vi "RotinaEnsaio.vi"() -> ()   [LabVIEW 2019]
uses:
  <vilib>/Platform/TimedLoop/XDataNode/timing_clust.ctl
  <vilib>/Platform/TimedLoop/XDataNode/nitl_modes.ctl
  <vilib>/Platform/TimedLoop/XDataNode/wakeup.ctl
  <vilib>/DAQmx/write.llb/DAQmx Write (Digital Bool 1Line 1Point).vi
  <vilib>/DAQmx/write.llb/DAQmx Write (Analog DBL 1Chan 1Samp).vi
  <vilib>/Analysis/5stat.llb/RMS (DBL).vi
  <vilib>/DAQmx/write.llb/DAQmx Write (Counter Frequency 1Chan 1Samp).vi
  <vilib>/DAQmx/create/channels.llb/DAQmx Create Channel (DO-Digital Output).vi
  <vilib>/DAQmx/miscellaneous.llb/DAQmx Fill In Error Info.vi
  FPGA_RW_Vars.vi
  <vilib>/DAQmx/create/channels.llb/DAQmx Create Channel (AO-Voltage-Basic).vi
  <vilib>/DAQmx/create/channels.llb/DAQmx Create Channel (CO-Pulse Generation-Frequency).vi
  <vilib>/DAQmx/configure/timing.llb/DAQmx Timing (Implicit).vi
  <vilib>/addons/control/pid/pid.llb/PID Advanced (DBL).vi
  <vilib>/Waveform/WDTFileIO.llb/ Write Waveform to File.vi
  <vilib>/Waveform/WDTFileIO.llb/ Write Waveforms to File (1D).vi
  <vilib>/Platform/TimedLoop/XDataNode/XDataNode.xnode
  <vilib>/addons/control/pid/NI_PID_pid.lvlib
  <vilib>/Analysis/NI_AALPro.lvlib
  <resource>/objmgr/daqmx.rc
  <vilib>/Platform/TimedLoop/XDataNode/XDNodeRunTimeDep.lvlib
  <vilib>/Analysis/NI_AALBase.lvlib
  <instrlib>/Yokogawa WT100 Series/Yokogawa WT100 Series.lvlib
panel:
  in  "error in 2":errorcluster caption="error in"
  in  "error in":errorcluster
  out "Tempo de Ensaio":string
  out "Erro Valv. Sucção":errorcluster
  out "Erro Pressão":errorcluster
  out "Erro Fluximetro":errorcluster
  in  "Ativar Compressor?":bool
  in  "Tab Control":T1(tab)
  in  "Temp. Suc. Auto?":bool
  in  "Setpoint T. Suc. [ºC]":dbl=60.0
  out "Duty Cycle da Resistência [%] 2":dbl min=0.0 max=100.0
  in  "DC da Resistência (Suc) [%]":dbl min=0.0 max=100.0
  out "GE Comp S [bar]":dbl
  out "GE Valv S [bar]":dbl
  out "RMS Inferior [g]":dbl
  out "RMS Bancada [g]":dbl
  out "RMS Superior [g]":dbl
  out "Grafico Vibração":T2(graph)
  out "Grafico Pressão":T3(graph)
  out "Tensão da válvula de sucção [V]":dbl min=0.0 max=100.0
  out "Duty Cycle da Resistência [%]":dbl min=0.0 max=100.0
  out "Setpoint da abertura da valvula":dbl=3720000.0
  out "Velocidade do motor de descarga":dbl
  in  "Tensão da válvula de sucção [V]":dbl=0.2 min=0.0 max=100.0
  out "Vazão Mássica [kg/h]":dbl
  in  "Ativar Ventilador?":bool=TRUE
  in  "P. Sucção Auto?":bool
  in  "Setpoint Sucção [bar]":dbl=0.626
  out "Descarga [bar]":dbl
  out "Sucção [bar]":dbl
  in  "Setpoint T. Desc. [ºC]":dbl=60.0
  in  "Temp. Desc. Auto?":bool
  out "Corrente RMS [A] (LEM)":dbl
  out "Descarga [ºC]":dbl
  out "Sucção [ºC]":dbl
  out "Grafico Temperatura":T4(graph)
  out "Bobina 2 [ºC]":dbl
  in  "DC da Resistência (Des) [%]":dbl min=0.0 max=100.0
  in  "Abertura da válvula de descarga":dbl=16000.0 format="%#_10f"
  in  "Velocidade do motor de descarga":dbl
  out "Grafico Corrente":T5(graph)
  out "Grafico Vazão":dbl(graph)
  out "Posição Atual da Válvula de Descarga":dbl format="%#_9f"
  out "Intermed [bar]":dbl
  in  "Vel. Valv. Desc. Auto?":bool=TRUE
  in  "P. Descarga Auto?":bool
  in  "Setpoint Descarga [bar]":dbl=7.616
  out "Abertura Atual da Válvula de Descarga":dbl format="%#_9f"
  out "Corrente RMS [A] (WT130)":dbl
  out "Tensão RMS [V] (WT130)":dbl
  out "Potência [W] (WT130)":dbl
  out "Corrente RMS [A] (TMCS)":dbl
  out "Bobina 1 [ºC]":dbl
  out "Tensão RMS [V] (DAQ)":dbl
  out "Corpo [ºC]":dbl
  out "Ambiente [ºC]":dbl
  out "Reservatório [ºC]":dbl
  in  "Unidade Pressão":T6(ring)
  in  "Eixo X":u16(ring) items=["Amostras", "Tempo [s]", "Tempo [min]", "Tempo [h]"]
  out "T.S. Auto?":bool
  in  "Ganhos - Temperatura Sucção":T7={"proportional gain (Kc)"=0.1, "integral time (Ti, min)"=30.0, "derivative time (Td, min)"=0.5} {"derivative time (Td, min)" format="%#_10g"; "integral time (Ti, min)" format="%#_10g"; "proportional gain (Kc)" format="%#_10g"}
  in  "Frequência PWM [Hz]":dbl=2.0 min=1e-12
  in  "Pasta do projeto":path=path "D:/Documentos/Amaciamento/Resultados/TESTE"
  out "dt - Leitura Temperatura [s]":dbl
  out "dt - At PressãoTemp/Le Pos":dbl
  out "dt - Leitura Fluxímetro [s]":dbl
  out "dt - Salvar dados [s]":dbl
  out "dt - Atualiza Gráficos [s]":dbl
  in  "Nome de Base do Arquivo - Geral":string="medicoesGerais"
  in  "Limite inferior da posição da válvula":dbl=3698950.0 format="%#_10f"
  out "T.D. Auto?":bool
  out "P. S. Auto?":bool
  out "P. D. Auto?":bool
  in  "Ganhos - Pressão de Descarga":T7={"proportional gain (Kc)"=-6000.0, "integral time (Ti, min)"=0.5, "derivative time (Td, min)"=0.0} {"derivative time (Td, min)" format="%#_10g"; "integral time (Ti, min)" format="%#_10g"; "proportional gain (Kc)" format="%#_10g"}
  out "Vel. M. Auto?":bool
  in  "Ganhos - Posição do motor":T7={"proportional gain (Kc)"=-0.27, "integral time (Ti, min)"=0.0, "derivative time (Td, min)"=0.0} {"derivative time (Td, min)" format="%#_10g"; "integral time (Ti, min)" format="%#_10g"; "proportional gain (Kc)" format="%#_10g"}
  in  "Ganhos - Pressão de Sucção":T7={"proportional gain (Kc)"=2.0, "integral time (Ti, min)"=0.2, "derivative time (Td, min)"=0.0} {"derivative time (Td, min)" format="%#_10g"; "integral time (Ti, min)" format="%#_10g"; "proportional gain (Kc)" format="%#_10g"}
  in  "Ganhos - Temperatura Descarga":T7={"proportional gain (Kc)"=0.1, "integral time (Ti, min)"=30.0, "derivative time (Td, min)"=0.5} {"derivative time (Td, min)" format="%#_10g"; "integral time (Ti, min)" format="%#_10g"; "proportional gain (Kc)" format="%#_10g"}
  in  "Limites de velocidade":T8={"Velocidade Máxima"=10000.0, "Velocidade Mínima"=-10000.0}
  in  "Nome de Base do Arquivo - Vibração":string="vib"
  in  "Nome de Base do Arquivo - Corrente":string="corr"
  out "dt - Controle Pressão [s]":dbl
  in  "Limite Superior DC Auto [%]":dbl=60.0 format="%#_13g"
  in  "Limite inferior - Válvula de sucção":dbl=0.18 format="%#_13g"
  in  "Nome de Base do Arquivo - Tensão":string="ten"
  out "G Temperaturas":T4(graph)
  out "G Pressão de Descarga":T9(graph)
  out "G Pressão de Sucção":T10(graph)
  out "G Corrente RMS":T5(graph)
  out "G Pressão Intermed":dbl(graph)
  out "G Vazão":dbl(graph)
  out "G Vel. do Motor da Válvula de Descarga":dbl(graph)
  out "G Posição do Encoder":T11(graph)
  out "G Tensão na válvula de Sucção":dbl(graph)
  out "Erro FPGA":errorcluster
  out "G Potência Yokogawa":dbl(graph)
  out "DC":dbl(graph)
  out "Error Out":errorcluster
  out "G Tensão Yokogawa":dbl(graph)
  out "Erro Motor":errorcluster
  out "error out":errorcluster
  out "Acc":dbl[](array[numeric])
  in  "STOP":bool
  in  "Limpar Gráficos":bool
  # "Isobutano (R600a):\n\n-23,3/54,4 -> 0,626/7,616\n-17,5/90    -> 0,8012/16,4073\n-10/100     -> 1,08127/19,8569\n\nR134a\n\n -23,3/54,4 -> 1,148/14,698"
  # "Pressão"
  # "Temperatura"
  # "Corrente"
  # "Vazão"
  # "Vibração"
  # "Controle Manual"
  # "Controle Aplicado"
  # "PID"
  # "Ranges"
  # "Arquivos"
  # "Resistência"
  # "Loops"
  # "Gráficos"
  # "Identificação de sistemas"
  # "Erros"
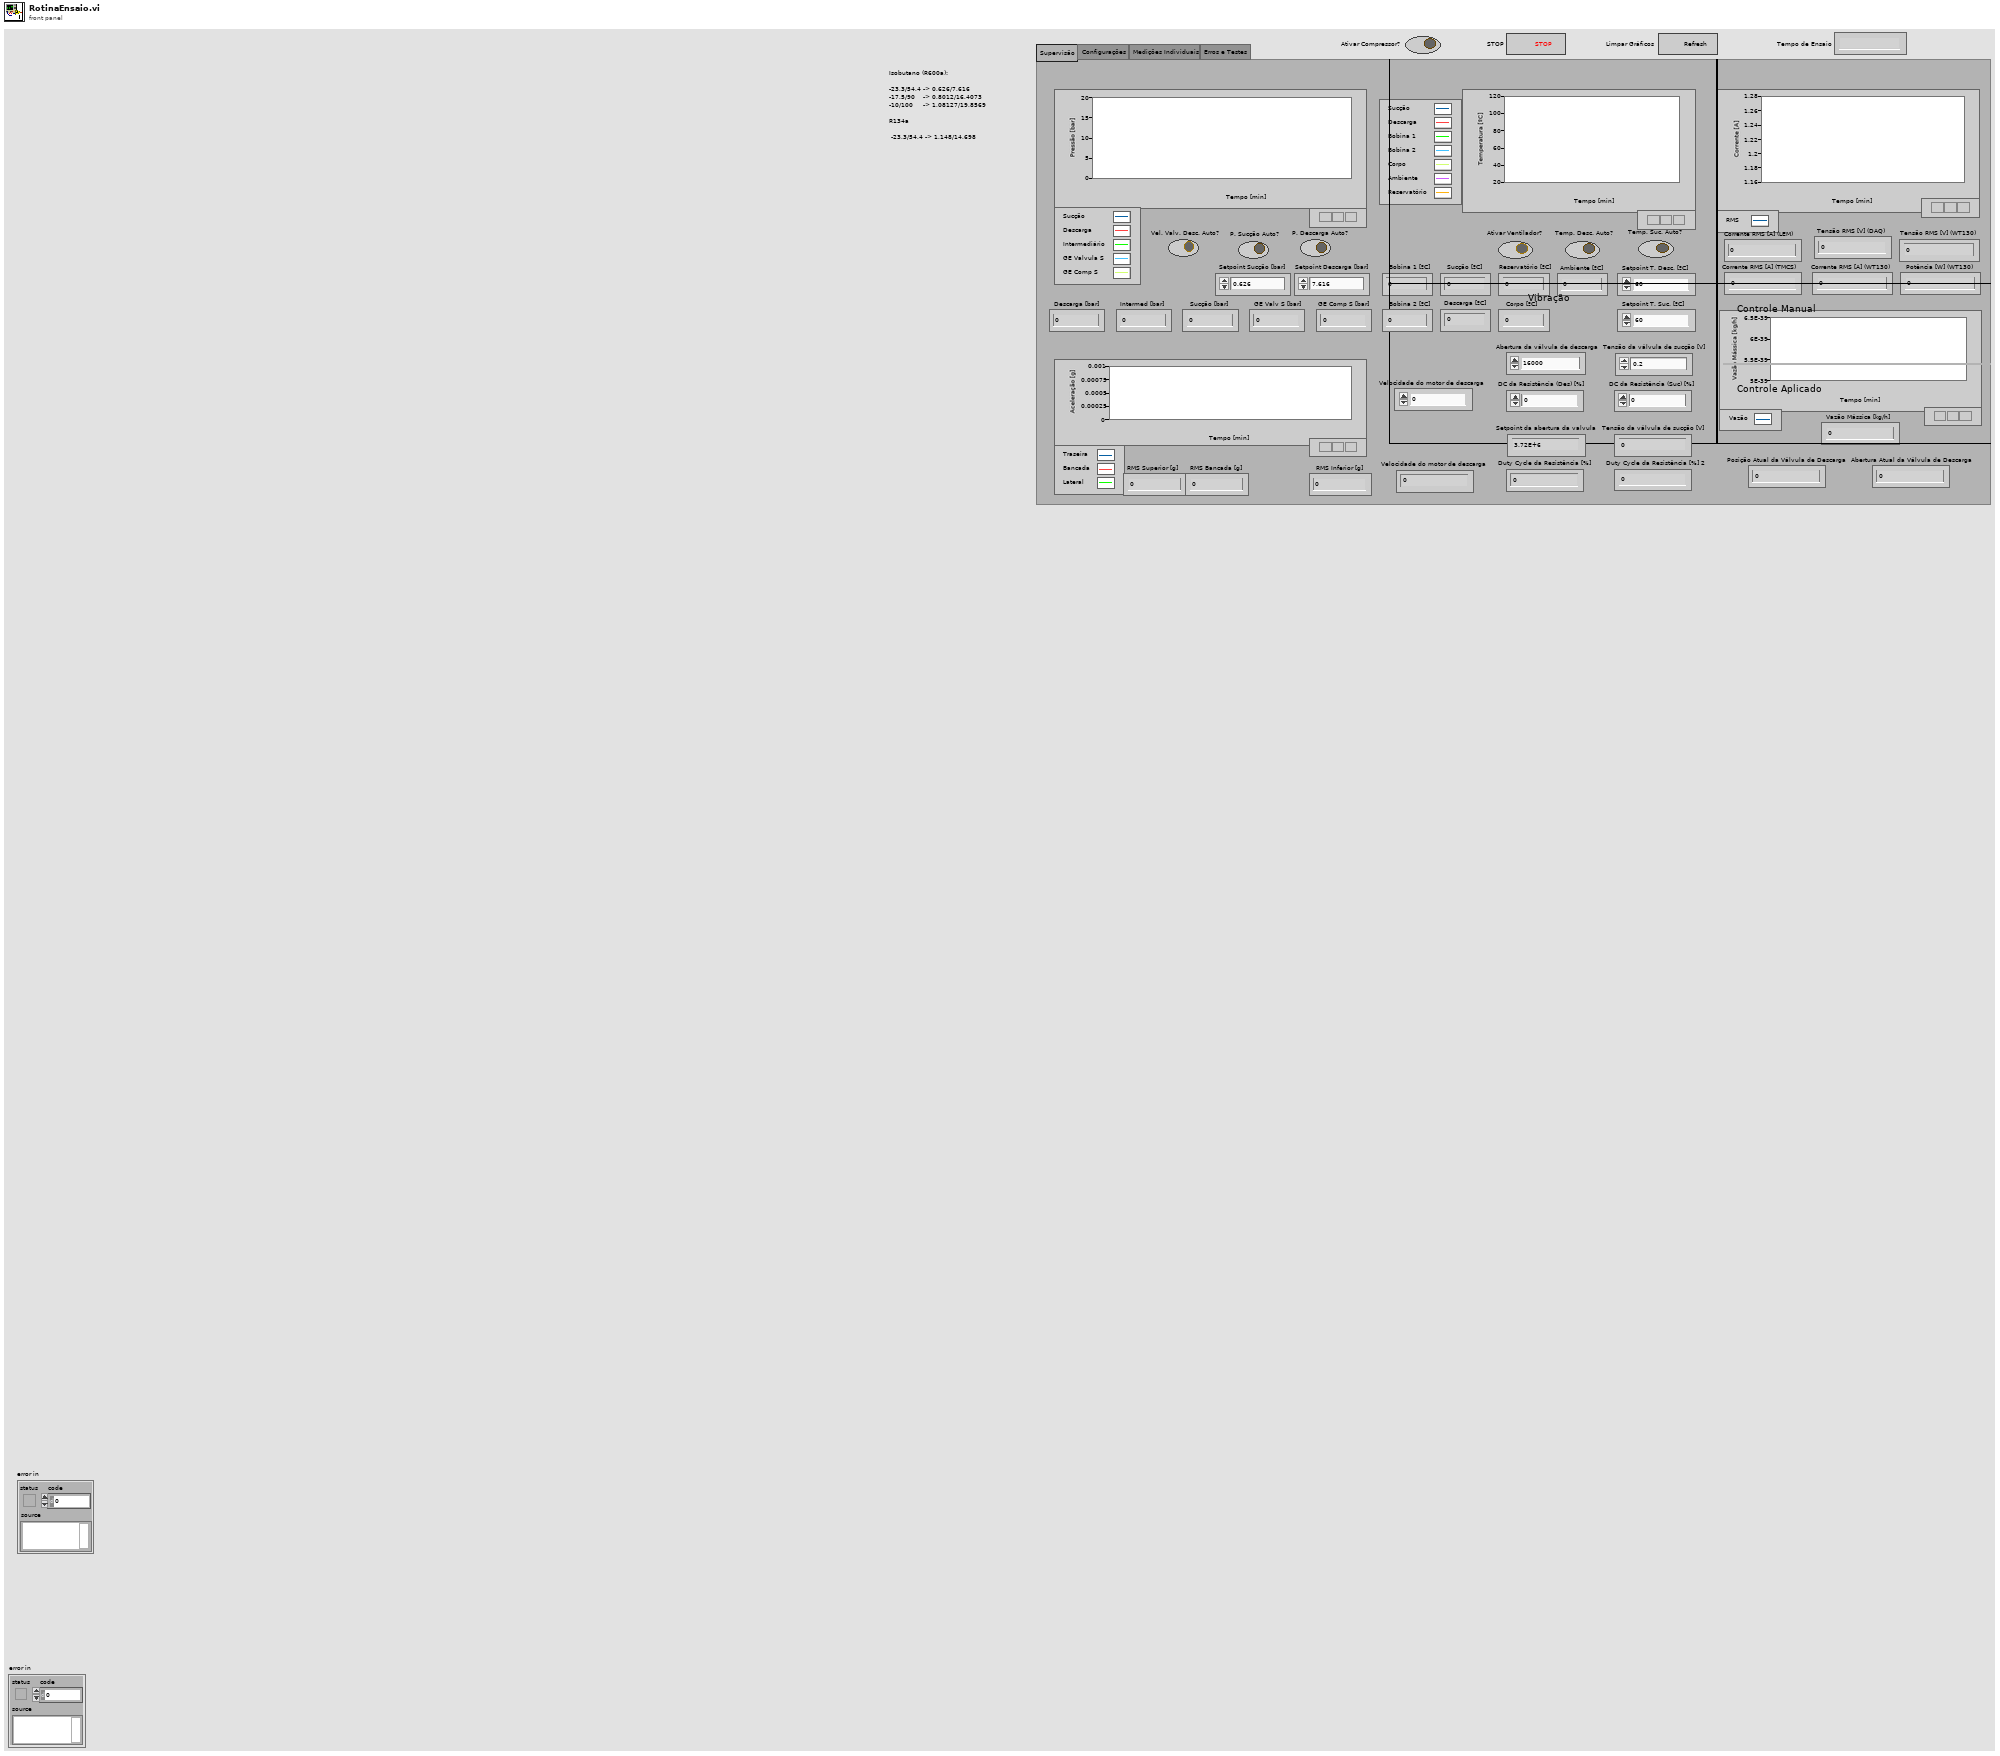
[diagram p1: front panel]
types:
  T1 = enum32{"Supervisão", "Configurações", "Medições Individuais", "Erros e Testes"}
  T2 = cluster{"Aceleração RMS Parede [g]":dbl, "Aceleração RMS Bancada [g]":dbl, "Aceleração RMS Corpo [g]":dbl}
  T3 = cluster{"Sucção [bar]":dbl, "Descarga [bar]":dbl, "Intermed [bar]":dbl, "GE Valv S [bar]":dbl, "GE Comp S [bar]":dbl}
  T4 = cluster{"Sucção [ºC]":dbl, "Descarga [ºC]":dbl, "Bobina 1 [ºC]":dbl, "Bobina 2 [ºC]":dbl, "Corpo [ºC]":dbl, "Ambiente [ºC]":dbl, "Reservatório [ºC]":dbl}
  T5 = cluster{"Corrente RMS [A]":dbl, "Corrente RMS [A]":dbl}
  T6 = enum16{"Pressão [bar]", "Temperatura R600 [ºC]", "Temperatura R134 [ºC]"}
  T7 = cluster{"proportional gain (Kc)":dbl, "integral time (Ti, min)":dbl, "derivative time (Td, min)":dbl}
  T8 = cluster{"Velocidade Máxima":dbl, "Velocidade Mínima":dbl}
  T9 = cluster{"Descarga Filtrada [bar]":dbl, "Setpoint Descarga [bar]":dbl}
  T10 = cluster{"Setpoint Sucção [bar]":dbl, "Sucção [bar]":dbl}
  T11 = cluster{"Abertura Atual da Válvula de Descarga":dbl, "Setpoint da abertura da valvula":dbl}
  T12 = cluster{"Acionador":tag, "Clock":tag, "Canal Analogico":tag, "Trigger":tag}
  T13 = cluster{"Sucção [bar]":dbl, "Descarga [bar]":dbl, "Intermed [bar]":dbl, "GE Valv S [bar]":dbl, "GE Comp S [bar]":dbl}[]
  T14 = cluster{"protocolStackName":string, "interfaceName":string, "portName":string, "baudrate":u32, "timeout":u32}
  T15 = cluster{"deviceName":string, "NodeID":u8, "velocity profile":cluster{"profileAcceleration":u32, "profileDeceleration":u32}}
  T16 = cluster{"Setpoint da posição da valvula":dbl, "Posição":dbl, "Setpoint Descarga [bar]":dbl}[]
  T17 = enum16{"open", "replace", "create", "open or create", "replace or create", "replace or create with confirmation"}
  T18 = typedef "XDNodeRunTimeDep.lvlib/timing_clust.ctl" = cluster{"Expected End [f-1]":u64, "Actual End [f-1]":u64, "Finished Late? [f-1]":bool, "Expected End [i-1]":u64, "Actual End [i-1]":u64, "Finished Late? [i-1]":bool, "Expected Start [i]":u64, "Actual Start [i]":u64, "Expected Start [f]":u64, "Actual Start [f]":u64, "Source Name":string, "Structure Name":string, "Period":i64, "Deadline":i64, "Offset":i64, "Start":i64, "Priority":i32, "Timeout":i32, "Mode":T19, "Wakeup Reason":T20, "Error":errorcluster, "Source Type":string, "Secondary Source Type":string, "Global End Time":u64, "Global Start Time":u64, "Frame Duration":u64, "Iteration Duration":u64, "Assigned CPU":i32, "I/O Scan Engine Mode":u32}
  T19 = typedef "XDNodeRunTimeDep.lvlib/nitl_modes.ctl" = enum32{"No Change", "Process missed periods, maintain original phase", "Discard missed periods, maintain original phase", "Process missed periods, ignore original phase", "Discard missed periods, ignore original phase"}
  T20 = typedef "XDNodeRunTimeDep.lvlib/wakeup.ctl" = enum32{"Normal", "Aborted", "Asynchronous wakeup", "Timing source error", "Timed loop error", "Timeout"}
  T21 = cluster{"Sucção [ºC]":dbl, "Descarga [ºC]":dbl, "Bobina 1 [ºC]":dbl, "Bobina 2 [ºC]":dbl, "Corpo [ºC]":dbl, "Ambiente [ºC]":dbl, "Reservatório [ºC]":dbl}[]
  T22 = cluster{"Sucção [bar]":dbl, "Descarga [bar]":dbl}[]
  T23 = typedef "xobjhandle.ctl" = u32
  T24 = cluster{"Task Analógico":refnum<k21>, "Task Clock":refnum<k21>, "Task Acionador":refnum<k21>, "Task Trigger":tag}
  T25 = typedef "Semaphore RefNum" = refnum<k1>
  T26 = cluster{"Vibration Lower (CH0)":waveform(dbl), "Vibration Dummy (CH1)":waveform(dbl), "Vibration Upper (CH2)":waveform(dbl)}
  T27 = cluster{"Voltage LEM (CH0)":waveform(dbl), "Voltage TMCS (CH2)":waveform(dbl)}
  T28 = cluster{"Temperature (CH0)":dbl, "Temperature (CH1)":dbl, "Temperature (CH2)":dbl, "Temperature (CH3)":dbl}
  T29 = cluster{"Corrente RMS [A] (LEM)":dbl, "Corrente RMS [A] (WT130)":dbl}
  T30 = cluster{"Descarga [bar]":dbl, "Setpoint Descarga [bar]":dbl}
  T31 = cluster{"GE Comp S [bar]":dbl, "Setpoint Sucção [bar]":dbl}
  T32 = cluster{"RMS Superior [g]":dbl, "RMS Bancada [g]":dbl, "RMS Inferior [g]":dbl}
  T33 = cluster{"output high":dbl, "Limite inferior - Válvula de sucção":dbl}
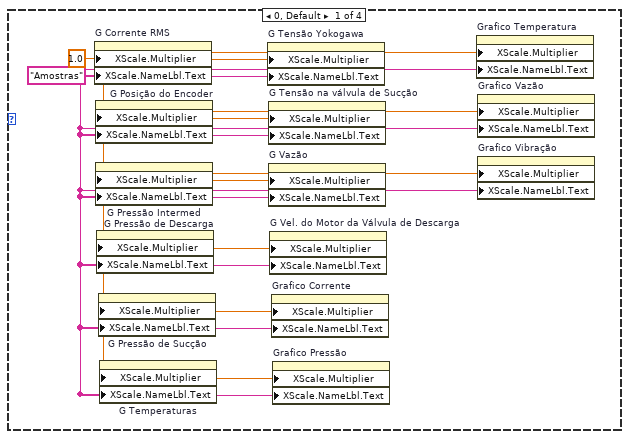
[diagram p2: hidden frame]
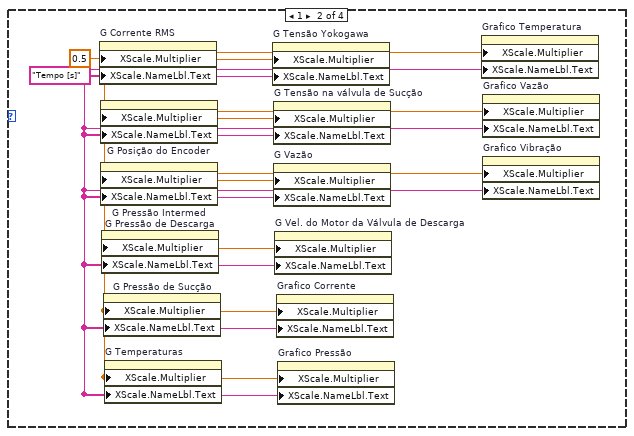
[diagram p3: hidden frame]
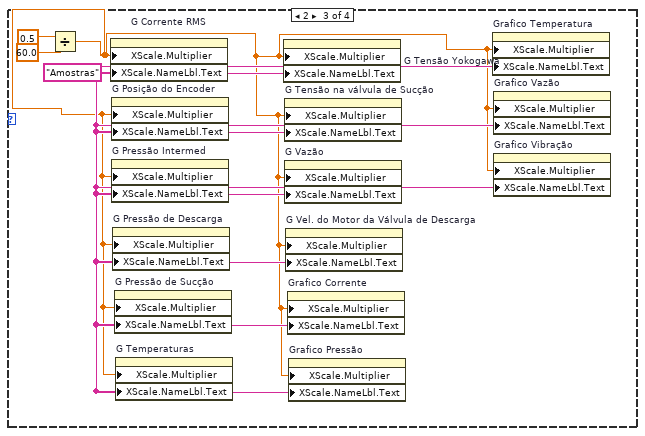
[diagram p4: hidden frame]
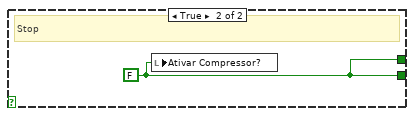
[diagram p13: hidden frame]
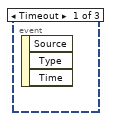
[diagram p14: hidden frame]
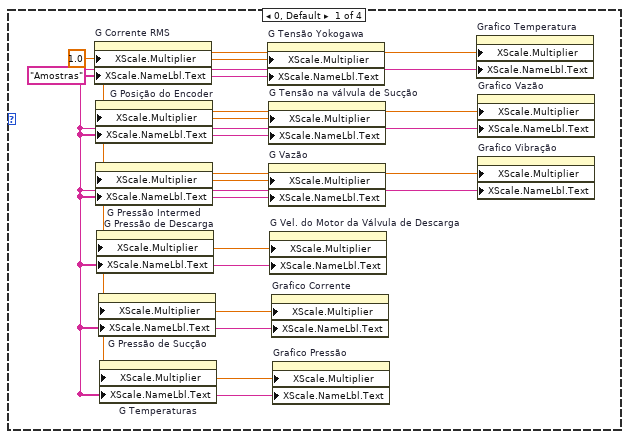
[diagram p15: hidden frame]
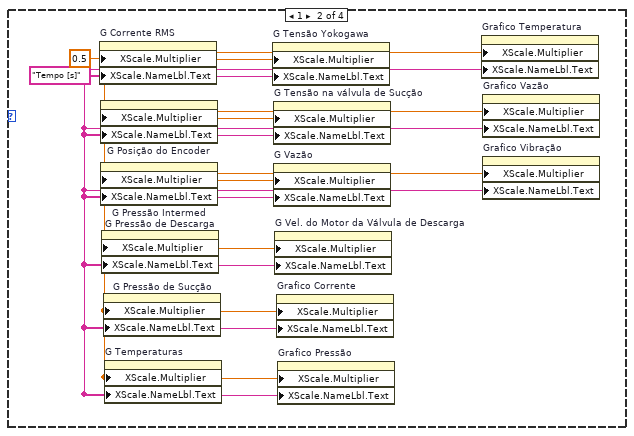
[diagram p16: hidden frame]
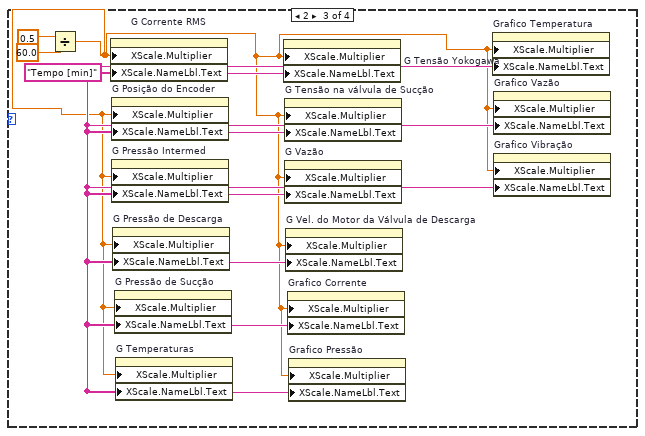
[diagram p17: hidden frame]
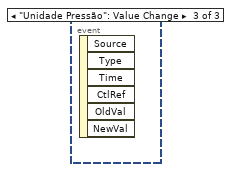
[diagram p18: hidden frame]
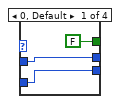
[diagram p20: hidden frame]
diagram:
  n1 = flat-sequence {
    tunnel: [w53] -> w3
    tunnel: [w51] -> w2
    tunnel: [w52] -> w1
    tunnel: [w99] -> w26
    tunnel: [w98] -> w23
    tunnel: [w88] -> w10
    tunnel: [w85] -> w7
    tunnel: [w83] -> w6
    tunnel: [w82] -> w5
    tunnel: [w81] -> w4
    tunnel: w3 -> [w83]
    tunnel: w2 -> [w82]
    tunnel: w1 -> [w81]
    tunnel: [w235] -> w49
    tunnel: [w193] -> w48
    tunnel: [w234] -> w47
    tunnel: [w242] -> w46
    tunnel: [w236] -> w45
    tunnel: [w243] -> w44
    tunnel: [w233] -> w43
    tunnel: [w244] -> w42
    tunnel: [w221] -> w41
    tunnel: [w245] -> w40
    tunnel: [w237] -> w39
    tunnel: [w222] -> w38
    tunnel: [w216] -> w37
    tunnel: [w214] -> w36
    tunnel: [w213] -> w35
    tunnel: [w212] -> w34
    tunnel: [w211] -> w33
    tunnel: [w123] -> w32
    tunnel: [w195] -> w31
    tunnel: [w192] -> w30
    tunnel: [w191] -> w29
    tunnel: [w196] -> w28
    tunnel: [w184] -> w27
    tunnel: w26 -> [w184]
    tunnel: [w183] -> w24
    tunnel: w23 -> [w183]
    tunnel: [w169] -> w21
    tunnel: [w168] -> w20
    tunnel: [w161] -> w17
    tunnel: [w138] -> w16
    tunnel: [w137] -> w15
    tunnel: [w122] -> w12
    tunnel: [w121] -> w11
    tunnel: w10 -> [w116]
    tunnel: [w120] -> w9
    tunnel: w7 -> [w115]
    tunnel: w6 -> [_]
    tunnel: w5 -> [w114]
    tunnel: w4 -> [w113]
    tunnel: w32 -> [w299]
    tunnel: w33 -> [w307]
    tunnel: w34 -> [w306]
    tunnel: w35 -> [w304]
    tunnel: w36 -> [w305]
    tunnel: w37 -> [w308]
    tunnel: w38 -> [w310]
    tunnel: w39 -> [w311]
    tunnel: w40 -> [w291]
    tunnel: w41 -> [w313]
    tunnel: w42 -> [w314]
    tunnel: w43 -> [w302]
    tunnel: w44 -> [w315]
    tunnel: w45 -> [w301]
    tunnel: w46 -> [w316]
    tunnel: w47 -> [w300]
    tunnel: w48 -> [w317]
    tunnel: w49 -> [w303]
    tunnel: w31 -> [w292]
    tunnel: w30 -> [w289]
    tunnel: w29 -> [w290]
    tunnel: w28 -> [w288]
    tunnel: w27 -> [w282]
    tunnel: [w282] -> w25
    tunnel: w24 -> [w280]
    tunnel: [w278] -> w22
    tunnel: w21 -> [w273]
    tunnel: w20 -> [w272]
    tunnel: [w271] -> w19
    tunnel: [w270] -> w18
    tunnel: w17 -> [w269]
    tunnel: w16 -> [w267]
    tunnel: w15 -> [w268]
    tunnel: [w268] -> w14
    tunnel: [w267] -> w13
    tunnel: w12 -> [w266]
    tunnel: w11 -> [w265]
    tunnel: w9 -> [w261]
    tunnel: [w261] -> w8
    tunnel: w25 -> [w910]
    tunnel: w22 -> [w911]
    tunnel: w19 -> [w906]
    tunnel: w18 -> [w905]
    tunnel: w14 -> [w896]
    tunnel: w13 -> [w895]
    tunnel: w8 -> [w894]
    frame #0 {
      n2 = flat-sequence {
        tunnel: [w74] -> w53
        tunnel: [w73] -> w52
        tunnel: [w67] -> w51
        frame #0 {
          n3 = Create Folder(path (use dialog)="Pasta do projeto") -> (created path=w71:path, error out=w70:errorcluster)  [unwired: 2 in, 1 out]
          n4 = case shown="No Error" w70 {
            tunnel: w71 -> [w75 _]
            tunnel: [w75 w76] -> w73
            tunnel: "Pasta do projeto" -> [_ w76]
            frame No Error {
            }
            frame Error {
            }
          }
          n5 = Concatenate Strings("Nome de Base do Arquivo - Geral", ".dat") -> (w74:string)
          n6 = Build Path(base path=w73, name or relative path=w74) -> (appended path=w67:path)
          n7 = call <vilib>:"Check if File or Folder Exists.vi"("path"=w67) -> ("file or folder exists?"=w66:bool)  [unwired: 8 in, 2 out]
          n8 = case shown="True" w66 {
            frame False {
            }
            frame True {
              n9 = Two Button Dialog(message="O caminho selecionado já contém arquivos de ensaios. Deseja continuar?", 1:"Continuar" ("F button name (\"Cancel\")"), 2:"Abortar" ("T button name (\"OK\")")) -> (T button?=w77:bool)
              n10 = Stop(stop? (T)=w77) -> ()
            }
          }
        }
      }
      n11 = case shown="3" "Eixo X" {
        frame 0, Default {
          w55 = "Amostras" ("X Scale.Name Label.Text")
          w54 = 1.0 ("X Scale.Offset and Multiplier:Multiplier")
          n12 = property on="G Corrente RMS" class="WFChart (strict)"("XScale.Multiplier"=w54, "XScale.NameLbl.Text"=w55) -> ()  [unwired: 2 in, 2 out]
          n13 = property on="G Posição do Encoder" class="WFChart (strict)"("XScale.Multiplier"=w54, "XScale.NameLbl.Text"=w55) -> ()  [unwired: 2 in, 2 out]
          n14 = property on="G Pressão Intermed" class="WFChart (strict)"("XScale.Multiplier"=w54, "XScale.NameLbl.Text"=w55) -> ()  [unwired: 2 in, 2 out]
          n15 = property on="G Pressão de Descarga" class="WFChart (strict)"("XScale.Multiplier"=w54, "XScale.NameLbl.Text"=w55) -> ()  [unwired: 2 in, 2 out]
          n16 = property on="G Pressão de Sucção" class="WFChart (strict)"("XScale.Multiplier"=w54, "XScale.NameLbl.Text"=w55) -> ()  [unwired: 2 in, 2 out]
          n17 = property on="G Temperaturas" class="WFChart (strict)"("XScale.Multiplier"=w54, "XScale.NameLbl.Text"=w55) -> ()  [unwired: 2 in, 2 out]
          n18 = property on="G Tensão Yokogawa" class="WFChart (strict)"("XScale.Multiplier"=w54, "XScale.NameLbl.Text"=w55) -> ()  [unwired: 2 in, 2 out]
          n19 = property on="G Tensão na válvula de Sucção" class="WFChart (strict)"("XScale.Multiplier"=w54, "XScale.NameLbl.Text"=w55) -> ()  [unwired: 2 in, 2 out]
          n20 = property on="G Vazão" class="WFChart (strict)"("XScale.Multiplier"=w54, "XScale.NameLbl.Text"=w55) -> ()  [unwired: 2 in, 2 out]
          n21 = property on="G Vel. do Motor da Válvula de Descarga" class="WFChart (strict)"("XScale.Multiplier"=w54, "XScale.NameLbl.Text"=w55) -> ()  [unwired: 2 in, 2 out]
          n22 = property on="Grafico Corrente" class="WFChart (strict)"("XScale.Multiplier"=w54, "XScale.NameLbl.Text"=w55) -> ()  [unwired: 2 in, 2 out]
          n23 = property on="Grafico Pressão" class="WFChart (strict)"("XScale.Multiplier"=w54, "XScale.NameLbl.Text"=w55) -> ()  [unwired: 2 in, 2 out]
          n24 = property on="Grafico Temperatura" class="WFChart (strict)"("XScale.Multiplier"=w54, "XScale.NameLbl.Text"=w55) -> ()  [unwired: 2 in, 2 out]
          n25 = property on="Grafico Vazão" class="WFChart (strict)"("XScale.Multiplier"=w54, "XScale.NameLbl.Text"=w55) -> ()  [unwired: 2 in, 2 out]
          n26 = property on="Grafico Vibração" class="WFChart (strict)"("XScale.Multiplier"=w54, "XScale.NameLbl.Text"=w55) -> ()  [unwired: 2 in, 2 out]
        }
        frame 1 {
          w57 = "Tempo [s]" ("X Scale.Name Label.Text")
          w56 = 0.5 ("X Scale.Offset and Multiplier:Multiplier")
          n27 = property on="G Corrente RMS" class="WFChart (strict)"("XScale.Multiplier"=w56, "XScale.NameLbl.Text"=w57) -> ()  [unwired: 2 in, 2 out]
          n28 = property on="G Posição do Encoder" class="WFChart (strict)"("XScale.Multiplier"=w56, "XScale.NameLbl.Text"=w57) -> ()  [unwired: 2 in, 2 out]
          n29 = property on="G Pressão Intermed" class="WFChart (strict)"("XScale.Multiplier"=w56, "XScale.NameLbl.Text"=w57) -> ()  [unwired: 2 in, 2 out]
          n30 = property on="G Pressão de Descarga" class="WFChart (strict)"("XScale.Multiplier"=w56, "XScale.NameLbl.Text"=w57) -> ()  [unwired: 2 in, 2 out]
          n31 = property on="G Pressão de Sucção" class="WFChart (strict)"("XScale.Multiplier"=w56, "XScale.NameLbl.Text"=w57) -> ()  [unwired: 2 in, 2 out]
          n32 = property on="G Temperaturas" class="WFChart (strict)"("XScale.Multiplier"=w56, "XScale.NameLbl.Text"=w57) -> ()  [unwired: 2 in, 2 out]
          n33 = property on="G Tensão Yokogawa" class="WFChart (strict)"("XScale.Multiplier"=w56, "XScale.NameLbl.Text"=w57) -> ()  [unwired: 2 in, 2 out]
          n34 = property on="G Tensão na válvula de Sucção" class="WFChart (strict)"("XScale.Multiplier"=w56, "XScale.NameLbl.Text"=w57) -> ()  [unwired: 2 in, 2 out]
          n35 = property on="G Vazão" class="WFChart (strict)"("XScale.Multiplier"=w56, "XScale.NameLbl.Text"=w57) -> ()  [unwired: 2 in, 2 out]
          n36 = property on="G Vel. do Motor da Válvula de Descarga" class="WFChart (strict)"("XScale.Multiplier"=w56, "XScale.NameLbl.Text"=w57) -> ()  [unwired: 2 in, 2 out]
          n37 = property on="Grafico Corrente" class="WFChart (strict)"("XScale.Multiplier"=w56, "XScale.NameLbl.Text"=w57) -> ()  [unwired: 2 in, 2 out]
          n38 = property on="Grafico Pressão" class="WFChart (strict)"("XScale.Multiplier"=w56, "XScale.NameLbl.Text"=w57) -> ()  [unwired: 2 in, 2 out]
          n39 = property on="Grafico Temperatura" class="WFChart (strict)"("XScale.Multiplier"=w56, "XScale.NameLbl.Text"=w57) -> ()  [unwired: 2 in, 2 out]
          n40 = property on="Grafico Vazão" class="WFChart (strict)"("XScale.Multiplier"=w56, "XScale.NameLbl.Text"=w57) -> ()  [unwired: 2 in, 2 out]
          n41 = property on="Grafico Vibração" class="WFChart (strict)"("XScale.Multiplier"=w56, "XScale.NameLbl.Text"=w57) -> ()  [unwired: 2 in, 2 out]
        }
        frame 2 {
          w61 = "Amostras" ("X Scale.Name Label.Text")
          n42 = Divide(x=0.5 ("X Scale.Offset and Multiplier:Multiplier"), y=60.0) -> (x/y=w58:dbl)
          n43 = property on="G Corrente RMS" class="WFChart (strict)"("XScale.Multiplier"=w58, "XScale.NameLbl.Text"=w61) -> ()  [unwired: 2 in, 2 out]
          n44 = property on="G Posição do Encoder" class="WFChart (strict)"("XScale.Multiplier"=w58, "XScale.NameLbl.Text"=w61) -> ()  [unwired: 2 in, 2 out]
          n45 = property on="G Pressão Intermed" class="WFChart (strict)"("XScale.Multiplier"=w58, "XScale.NameLbl.Text"=w61) -> ()  [unwired: 2 in, 2 out]
          n46 = property on="G Pressão de Descarga" class="WFChart (strict)"("XScale.Multiplier"=w58, "XScale.NameLbl.Text"=w61) -> ()  [unwired: 2 in, 2 out]
          n47 = property on="G Pressão de Sucção" class="WFChart (strict)"("XScale.Multiplier"=w58, "XScale.NameLbl.Text"=w61) -> ()  [unwired: 2 in, 2 out]
          n48 = property on="G Temperaturas" class="WFChart (strict)"("XScale.Multiplier"=w58, "XScale.NameLbl.Text"=w61) -> ()  [unwired: 2 in, 2 out]
          n49 = property on="G Tensão Yokogawa" class="WFChart (strict)"("XScale.Multiplier"=w58, "XScale.NameLbl.Text"=w61) -> ()  [unwired: 2 in, 2 out]
          n50 = property on="G Tensão na válvula de Sucção" class="WFChart (strict)"("XScale.Multiplier"=w58, "XScale.NameLbl.Text"=w61) -> ()  [unwired: 2 in, 2 out]
          n51 = property on="G Vazão" class="WFChart (strict)"("XScale.Multiplier"=w58, "XScale.NameLbl.Text"=w61) -> ()  [unwired: 2 in, 2 out]
          n52 = property on="G Vel. do Motor da Válvula de Descarga" class="WFChart (strict)"("XScale.Multiplier"=w58, "XScale.NameLbl.Text"=w61) -> ()  [unwired: 2 in, 2 out]
          n53 = property on="Grafico Corrente" class="WFChart (strict)"("XScale.Multiplier"=w58, "XScale.NameLbl.Text"=w61) -> ()  [unwired: 2 in, 2 out]
          n54 = property on="Grafico Pressão" class="WFChart (strict)"("XScale.Multiplier"=w58, "XScale.NameLbl.Text"=w61) -> ()  [unwired: 2 in, 2 out]
          n55 = property on="Grafico Temperatura" class="WFChart (strict)"("XScale.Multiplier"=w58, "XScale.NameLbl.Text"=w61) -> ()  [unwired: 2 in, 2 out]
          n56 = property on="Grafico Vazão" class="WFChart (strict)"("XScale.Multiplier"=w58, "XScale.NameLbl.Text"=w61) -> ()  [unwired: 2 in, 2 out]
          n57 = property on="Grafico Vibração" class="WFChart (strict)"("XScale.Multiplier"=w58, "XScale.NameLbl.Text"=w61) -> ()  [unwired: 2 in, 2 out]
        }
        frame 3 {
          w62 = "Amostras" ("X Scale.Name Label.Text")
          n58 = Divide(x=0.5 ("X Scale.Offset and Multiplier:Multiplier"), y=3600.0) -> (x/y=w65:dbl)
          n59 = property on="G Corrente RMS" class="WFChart (strict)"("XScale.Multiplier"=w65, "XScale.NameLbl.Text"=w62) -> ()  [unwired: 2 in, 2 out]
          n60 = property on="G Posição do Encoder" class="WFChart (strict)"("XScale.Multiplier"=w65, "XScale.NameLbl.Text"=w62) -> ()  [unwired: 2 in, 2 out]
          n61 = property on="G Pressão Intermed" class="WFChart (strict)"("XScale.Multiplier"=w65, "XScale.NameLbl.Text"=w62) -> ()  [unwired: 2 in, 2 out]
          n62 = property on="G Pressão de Descarga" class="WFChart (strict)"("XScale.Multiplier"=w65, "XScale.NameLbl.Text"=w62) -> ()  [unwired: 2 in, 2 out]
          n63 = property on="G Pressão de Sucção" class="WFChart (strict)"("XScale.Multiplier"=w65, "XScale.NameLbl.Text"=w62) -> ()  [unwired: 2 in, 2 out]
          n64 = property on="G Temperaturas" class="WFChart (strict)"("XScale.Multiplier"=w65, "XScale.NameLbl.Text"=w62) -> ()  [unwired: 2 in, 2 out]
          n65 = property on="G Tensão Yokogawa" class="WFChart (strict)"("XScale.Multiplier"=w65, "XScale.NameLbl.Text"=w62) -> ()  [unwired: 2 in, 2 out]
          n66 = property on="G Tensão na válvula de Sucção" class="WFChart (strict)"("XScale.Multiplier"=w65, "XScale.NameLbl.Text"=w62) -> ()  [unwired: 2 in, 2 out]
          n67 = property on="G Vazão" class="WFChart (strict)"("XScale.Multiplier"=w65, "XScale.NameLbl.Text"=w62) -> ()  [unwired: 2 in, 2 out]
          n68 = property on="G Vel. do Motor da Válvula de Descarga" class="WFChart (strict)"("XScale.Multiplier"=w65, "XScale.NameLbl.Text"=w62) -> ()  [unwired: 2 in, 2 out]
          n69 = property on="Grafico Corrente" class="WFChart (strict)"("XScale.Multiplier"=w65, "XScale.NameLbl.Text"=w62) -> ()  [unwired: 2 in, 2 out]
          n70 = property on="Grafico Pressão" class="WFChart (strict)"("XScale.Multiplier"=w65, "XScale.NameLbl.Text"=w62) -> ()  [unwired: 2 in, 2 out]
          n71 = property on="Grafico Temperatura" class="WFChart (strict)"("XScale.Multiplier"=w65, "XScale.NameLbl.Text"=w62) -> ()  [unwired: 2 in, 2 out]
          n72 = property on="Grafico Vazão" class="WFChart (strict)"("XScale.Multiplier"=w65, "XScale.NameLbl.Text"=w62) -> ()  [unwired: 2 in, 2 out]
          n73 = property on="Grafico Vibração" class="WFChart (strict)"("XScale.Multiplier"=w65, "XScale.NameLbl.Text"=w62) -> ()  [unwired: 2 in, 2 out]
        }
      }
    }
    frame #1 {
      w86 = FALSE ("Reading?")
      w94 = FALSE ("P. Sucção Auto?")
      w93 = 0.0 ("Duty Cycle da Resistência [%]")
      # "Inicializa Timer Segurança"
      n74 = global write "FPGA_RW_Vars.vi" "Error Out"(errorcluster {"status"=FALSE, "code"=0, "source"=""} ("Error Out")) -> ()
      n75 = global write "FPGA_RW_Vars.vi" "Reading?"(w86) -> ()
      n76 = global write "FPGA_RW_Vars.vi" "Stop"(w86) -> ()
      n77 = call <vilib>:"Application Directory.vi"() -> ("Application Directory"=w92:path)
      n78 = call-poly <vilib>:"DAQmx Create Virtual Channel.vi"("lines"=tag "Dev1/port1/line5") -> ("task out"=w104:refnum<k21>, "error out"=w105:errorcluster)  [unwired: 13 in]
      n79 = Build Path(base path=w92, name or relative path="PC_Consumer_DMA.vi") -> (appended path=w90:path)
      n80 = call-poly <vilib>:"DAQmx Create Virtual Channel.vi"("lines"=tag "Dev1/port1/line4") -> ("task out"=w102:refnum<k21>, "error out"=w101:errorcluster)  [unwired: 13 in]
      n81 = local write "P. Descarga Auto?"(w94) -> ()
      n82 = local write "DC da Resistência (Des) [%]"(w93) -> ()
      n83 = local write "DC da Resistência (Suc) [%]"(w93) -> ()
      n84 = local write "P. Sucção Auto?"(w94) -> ()
      n85 = call <vilib>:"DAQmx Start Task.vi"("task/channels in"=w104, "error in"=w105) -> ("task out"=w103:refnum<k21>)  [unwired: 12 in, 1 out]
      n86 = Open VI Reference(type specifier VI Refnum (for type only)=refnum<vi> refnum, vi path=w90, options=128) -> (vi reference=w88:refnum<vi>, error out=w85:errorcluster)  [unwired: 3 in]
      n87 = call <vilib>:"DAQmx Start Task.vi"("task/channels in"=w102, "error in"=w101) -> ("task out"=w100:refnum<k21>)  [unwired: 12 in, 1 out]
      n88 = call-poly <vilib>:"DAQmx Write.vi"("task/channels in"=w103, "data"=FALSE) -> ("task out"=w99:refnum<k21>)  [unwired: 11 in, 2 out]
      n89 = call-poly <vilib>:"DAQmx Write.vi"("task/channels in"=w100, "data"=TRUE) -> ("task out"=w98:refnum<k21>)  [unwired: 11 in, 2 out]
      n90 = Wait (ms)(milliseconds to wait=u32 2000) -> ()  [unwired: 1 out]
    }
    frame #2 {
      w119 = T21 [] ("History Data")
      w132 = 10123 items=["Finite Samples"=10178, "Continuous Samples"=10123, "Hardware Timed Single Point"=12522] ("sample mode")
      w149 = "Dev1/ao2"  # physical channel
      w147 = TRUE  # auto cleanup
      w139 = 10083 items=["Default"=-1, "RSE"=10083, "Differential"=10106, "Pseudodifferential"=12529]  # output terminal configuration
      w153 = 10348 items=["Volts"=10348, "From Custom Scale"=10065]  # units
      w154 = "VoltageOut"  # channel name
      w155 = ""  # custom scale name
      w141 = -5.0  # minimum value
      w140 = 5.0  # maximum value
      w156 = "Dev1/ao1"  # physical channel
      w158 = TRUE  # auto cleanup
      w174 = u16 0  # Auto range
      w179 = FALSE  # not hrm
      w182 = u16 0  # Normal Mode
      w191 = u32[] [7, 2]  # DPS NodeID
      w202 = 10123 items=["Finite Samples"=10178, "Continuous Samples"=10123, "Hardware Timed Single Point"=12522] ("sample mode")
      w215 = dbl[] [] ("History Data")
      w167 = T22 [] ("History Data")
      w221 = refnum<visa-resource-name> "COM3" ("VISA resource")
      w244 = u16 1 ("Endereço slave")
      # "Inicialização alimentação do transdutor de corrente (TMCS)"
      # "Inicialização ventilador"
      # "Inicialização compressor"
      # "Inicialização das Resistências"
      # "Inicia leitura do Fluxímetro"
      # "Inicia zerando os gráficos"
      # "Inicializa Equipamentos"
      n91 = local read "DC da Resistência (Suc) [%]"() -> (w108:dbl)
      n92 = local read "DC da Resistência (Des) [%]"() -> (w109:dbl)
      n93 = call-by-ref "Start Asynchronous Call"(reference=w116, error in=w115) -> (reference out=w117:refnum<vi>, error out=w118:errorcluster)  [unwired: 12 in]
      n94 = call <vilib>:"DAQmx Create Task.vi"("auto cleanup"=w147, "error in"="error in 2") -> ("task out"=w148:refnum<k21>, "error out"=w146:errorcluster)  [unwired: 12 in]
      n95 = Build Path(base path=w113, name or relative path="vibracao\\") -> (appended path=w223:path)
      n96 = Build Path(base path=w113, name or relative path="corrente\\") -> (appended path=w217:path)
      n97 = Build Path(base path=w113, name or relative path="tensao\\") -> (appended path=w165:path)
      n98 = call <vilib>:"DAQmx Create Task.vi"("auto cleanup"=w158, "error in"="error in") -> ("task out"=w157:refnum<k21>, "error out"=w159:errorcluster)  [unwired: 12 in]
      n99 = property on="Grafico Vibração" class="WFChart (strict)"("History Data"=T16 []) -> ()  [unwired: 2 in, 2 out]
      n100 = Divide(x=w108, y=100.0) -> (x/y=w128:dbl)
      n101 = Divide(x=w109, y=100.0) -> (x/y=w206:dbl)
      n102 = property on="Grafico Temperatura" class="WFChart (strict)"("History Data"=w119) -> ()  [unwired: 2 in, 2 out]
      n103 = property on="G Temperaturas" class="WFChart (strict)"("History Data"=w119) -> ()  [unwired: 2 in, 2 out]
      n104 = property on="Grafico Pressão" class="WFChart (strict)"("History Data"=T13 []) -> ()  [unwired: 2 in, 2 out]
      n105 = local read "Frequência PWM [Hz]"() -> (w123:dbl)
      n106 = Create Folder(path (use dialog)=w223) -> (created path=w224:path, error out=w226:errorcluster)  [unwired: 2 in, 1 out]
      n107 = Create Folder(path (use dialog)=w165) -> (created path=w164:path, error out=w162:errorcluster)  [unwired: 2 in, 1 out]
      n108 = Create Folder(path (use dialog)=w217) -> (created path=w218:path, error out=w220:errorcluster)  [unwired: 2 in, 1 out]
      n109 = global write "FPGA_RW_Vars.vi" "Error Out"(w118) -> ()
      n110 = In Range and Coerce(upper limit=0.99999988 ("output high"), x=w128, lower limit=1.19209297e-07 ("output low")) -> (coerced(x)=w124:dbl)  [unwired: 1 out]
      n111 = In Range and Coerce(upper limit=0.99999988 ("output high"), x=w206, lower limit=1.19209297e-07 ("output low")) -> (coerced(x)=w210:dbl)  [unwired: 1 out]
      n112 = case shown="No Error" w226 {
        tunnel: w224 -> [w259 _]
        tunnel: [w259 w260] -> w222
        tunnel: w223 -> [_ w260]
        frame No Error {
        }
        frame Error {
        }
      }
      n113 = case shown="Error" w220 {
        tunnel: w218 -> [w257 _]
        tunnel: [w257 w258] -> w216
        tunnel: w217 -> [_ w258]
        frame No Error {
        }
        frame Error {
        }
      }
      n114 = case shown="No Error" w162 {
        tunnel: w164 -> [w252 _]
        tunnel: [w252 w253] -> w161
        tunnel: w165 -> [_ w253]
        frame No Error {
        }
        frame Error {
        }
      }
      n115 = call <instrlib>:"Initialize.vi"("error in (no error)"=errorcluster {"status"=FALSE, "code"=0, "source"=""}, "VISA resource name"=refnum<visa-resource-name> "GPIB0::1::INSTR") -> ("error out"=w172:errorcluster, "VISA resource name out"=w171:refnum<visa-resource-name>)  [unwired: 8 in]
      n116 = while {
        tunnel: w117 -> [w251]
        tunnel: [w251] -> w120
        tunnel: w118 -> [w247]
        stop <- w248 stop-if-true
        # "Espera até que a medição FPGA esteja disponível"
        n117 = global read "FPGA_RW_Vars.vi" "Reading?"() -> (w250:bool)
        n118 = global read "FPGA_RW_Vars.vi" "Error Out"() -> (w246:errorcluster)
        n119 = local read "STOP"() -> (w249:bool)
        n120 = Compound Arithmetic op=OR(w250, w249, w247, w246) -> (w248:bool)
      }
      n121 = call-poly <vilib>:"DAQmx Create Virtual Channel.vi"("frequency"=w123, "duty cycle"=w124, "counter"=tag "Dev1/ctr2") -> ("task out"=w135:refnum<k21>, "error out"=w136:errorcluster)  [unwired: 11 in]
      n122 = call-poly <vilib>:"DAQmx Create Virtual Channel.vi"("frequency"=w123, "duty cycle"=w210, "counter"=tag "Dev1/ctr3") -> ("task out"=w199:refnum<k21>, "error out"=w198:errorcluster)  [unwired: 11 in]
      n123 = call "intializeCAN_EPOS+DPS.vi"("DPS NodeID"=w191, "EPOS Settings"=T15 {"deviceName"="EPOS2", "NodeID"=8, "velocity profile"={"profileAcceleration"=1000, "profileDeceleration"=1000}}, "CAN Settings"=T14 {"protocolStackName"="CANopen", "interfaceName"="NI_PCI-CAN 0", "portName"="CAN0", "baudrate"=500000, "timeout"=1000}) -> ("DPS error out"=w187:errorcluster, "EPOS error out"=w186:errorcluster, "ObjHandle out"=w192:T23, "axis out"=w193:cluster{"keyHandle":u32, "nodeId":u16})  [unwired: 1 in]
      n124 = property on="G Vazão" class="WFChart (strict)"("History Data"=w215) -> ()  [unwired: 2 in, 2 out]
      n125 = call <instrlib>:"Config Mode.vi"("error in (no error)"=w172, "Mode (0: RMS)"=w182, "VISA resource name"=w171) -> ("error out"=w181:errorcluster, "VISA resource name out"=w180:refnum<visa-resource-name>)  [unwired: 7 in]
      n126 = call <instrlib>:"Config Harmonics.vi"("error in (no error)"=w181, "On/Off (F: Off)"=w179, "VISA resource name"=w180) -> ("error out"=w178:errorcluster, "VISA resource name out"=w177:refnum<visa-resource-name>)  [unwired: 7 in]
      n127 = property class="DAQmx Channel"(reference=w135, error in=w136, "CO.Pulse.Term"=tag "/Dev1/PFI3") -> (reference out=w130:refnum<k21>, error out=w134:errorcluster)
      n128 = property on="G Pressão Intermed" class="WFChart (strict)"("History Data"=w215) -> ()  [unwired: 2 in, 2 out]
      n129 = property on="Grafico Vazão" class="WFChart (strict)"("History Data"=w215) -> ()  [unwired: 2 in, 2 out]
      n130 = property on="G Tensão Yokogawa" class="WFChart (strict)"("History Data"=w215) -> ()  [unwired: 2 in, 2 out]
      n131 = property on="G Vel. do Motor da Válvula de Descarga" class="WFChart (strict)"("History Data"=w215) -> ()  [unwired: 2 in, 2 out]
      n132 = property on="G Tensão na válvula de Sucção" class="WFChart (strict)"("History Data"=w215) -> ()  [unwired: 2 in, 2 out]
      n133 = property on="G Potência Yokogawa" class="WFChart (strict)"("History Data"=w215) -> ()  [unwired: 2 in, 2 out]
      n134 = property class="DAQmx Channel"(reference=w199, error in=w198, "CO.Pulse.Term"=tag "/Dev1/PFI2") -> (reference out=w204:refnum<k21>, error out=w200:errorcluster)
      n135 = property on="G Pressão de Sucção" class="WFChart (strict)"("History Data"=w167) -> ()  [unwired: 2 in, 2 out]
      n136 = property on="G Pressão de Descarga" class="WFChart (strict)"("History Data"=w167) -> ()  [unwired: 2 in, 2 out]
      n137 = property on="G Posição do Encoder" class="WFChart (strict)"("History Data"=w167) -> ()  [unwired: 2 in, 2 out]
      n138 = call-poly <vilib>:"DAQmx Create Virtual Channel.vi"("task in"=w148, "maximum value"=w140, "minimum value"=w141, "output terminal configuration"=w139, "physical channels"=w149, "error in"=w146) -> ("task out"=w143:refnum<k21>, "error out"=w142:errorcluster)  [unwired: 8 in]
      n139 = property on="G Corrente RMS" class="WFChart (strict)"("History Data"=w167) -> ()  [unwired: 2 in, 2 out]
      n140 = property on="Grafico Corrente" class="WFChart (strict)"("History Data"=w167) -> ()  [unwired: 2 in, 2 out]
      n141 = call-poly <vilib>:"DAQmx Create Virtual Channel.vi"("task in"=w157, "maximum value"=w140, "minimum value"=w141, "output terminal configuration"=w139, "physical channels"=w156, "name to assign"=w154, "units"=w153, "error in"=w159, "custom scale name"=w155) -> ("task out"=w152:refnum<k21>, "error out"=w150:errorcluster)  [unwired: 5 in]
      n142 = call <instrlib>:"Config Voltage Range.vi"("error in (no error)"=w178, "Range (6: 600V)"=w174, "VISA resource name"=w177) -> ("error out"=w176:errorcluster, "VISA resource name out"=w175:refnum<visa-resource-name>)  [unwired: 7 in]
      n143 = Or(x=w186, y=w187) -> (x .or. y?=w188:bool)
      n144 = call <instrlib>:"Config Current Range.vi"("error in (no error)"=w176, "Range (6: 20A)"=w174, "VISA resource name"=w175) -> ("error out"=w168:errorcluster, "VISA resource name out"=w169:refnum<visa-resource-name>)  [unwired: 7 in]
      n145 = case shown="True" w188 {
        tunnel: w193 -> [_ w255]
        tunnel: w192 -> [_ w254]
        frame False {
        }
        frame True {
          n146 = Unbundle By Name(w255) -> ("keyHandle"=w256:u32)
          n147 = call <vilib>:"ncClose.vi"("ObjHandle in"=w254) -> ()  [unwired: 2 in, 1 out]
          n148 = call <instrlib>:"VCS Close Device.vi"("keyHandle in"=w256) -> ()  [unwired: 10 in, 1 out]
        }
      }
      n149 = call-poly <vilib>:"DAQmx Write.vi"("task/channels in"=w143, "data"=2.5, "error in"=w142) -> ("task out"=w138:refnum<k21>)  [unwired: 10 in, 2 out]
      n150 = call-poly <vilib>:"DAQmx Create Virtual Channel.vi"("lines"=tag "Dev1/port1/line0") -> ("task out"=w232:refnum<k21>, "error out"=w231:errorcluster)  [unwired: 13 in]
      n151 = call-poly <vilib>:"DAQmx Write.vi"("task/channels in"=w152, "data"=5.0, "error in"=w150) -> ("task out"=w137:refnum<k21>)  [unwired: 10 in, 2 out]
      n152 = call-poly <vilib>:"DAQmx Create Virtual Channel.vi"("lines"=tag "Dev1/port1/line1") -> ("task out"=w229:refnum<k21>, "error out"=w228:errorcluster)  [unwired: 13 in]
      n153 = Array To Spreadsheet String(array=string[] ["Tempo [s]", "Temperatura Bobina 1 [ºC]", "Temperatura Bobina 2 [ºC]", "Temperatura Sucção [ºC]", "Temperatura Descarga [ºC]", "Pressão Sucção [bar]", "Pressão Descarga [bar]", "Pressão Intermediária [bar]", "Setpoint da Abertura da Válvula [Passos]", "Abertura da válvula [Passos]", "Limite da válvula [Passos]", "Tensão da válvula de sucção [V]", "Corrente RMS [A]", "Compressor Ativado", "Aceleração RMS Inferior Corpo [g]", "Aceleração RMS Bancada [g]", "Aceleração RMS Superior Corpo [g]", "Vazão Mássica [kg/h]", "Duty Cycle Descarga [%]", "Pressão Sucção Válvula (DPS) [bar]", "Pressão Sucção Compressor (DPS) [bar]", "Corrente Yokogawa [A]", "Tensão Yokogawa [V]", "Potência Yokogawa [W]", "Corrente TMCS [A]", "Tensão DAQ [V]", "Temperatura Corpo [ºC]", "Temperatura Ambiente [ºC]", "Temperatura Reservatório [ºC]"], 3:"%s" ("format string")) -> (spreadsheet string=w241:string)  [unwired: 1 in]
      n154 = call-poly <vilib>:"DAQmx Timing.vi"("task/channels in"=w130, "sample mode"=w132, "error in"=w134) -> ("task out"=w131:refnum<k21>, "error out"=w129:errorcluster)  [unwired: 11 in]
      n155 = call-poly <vilib>:"DAQmx Timing.vi"("task/channels in"=w204, "sample mode"=w202, "error in"=w200) -> ("task out"=w203:refnum<k21>, "error out"=w205:errorcluster)  [unwired: 11 in]
      n156 = call <vilib>:"DAQmx Start Task.vi"("task/channels in"=w232, "error in"=w231) -> ("task out"=w235:refnum<k21>, "error out"=w233:errorcluster)  [unwired: 12 in]
      n157 = call <vilib>:"DAQmx Start Task.vi"("task/channels in"=w229, "error in"=w228) -> ("task out"=w214:refnum<k21>, "error out"=w213:errorcluster)  [unwired: 12 in]
      n158 = call <vilib>:"High Resolution Relative Seconds.vi"() -> ("relative seconds"=w245:dbl)
      n159 = Open/Create/Replace File(file path (use dialog)=w114, operation (0:open)=T17."replace or create with confirmation") -> (refnum out=w240:refnum<file>)  [unwired: 4 in, 2 out]
      n160 = call "FluxCreate.vi"("Endereço slave"=w244, "Recurso VISA"=w221) -> ("Error Out"=w243:errorcluster, "Master Out"=w242:refnum<class "Modbus Master.lvclass">)
      n161 = call <vilib>:"DAQmx Start Task.vi"("task/channels in"=w131, "error in"=w129) -> ("task out"=w122:refnum<k21>, "error out"=w121:errorcluster)  [unwired: 12 in]
      n162 = call "Encoder Init.vi"("Portas"=T12 {"Acionador"="Dev1/port0/line7", "Clock"="Dev1/ctr0", "Canal Analogico"="Dev1/ai22", "Trigger"="/Dev1/PFI11"}) -> ("Task Out"=w212:T24, "error out"=w211:errorcluster)  [unwired: 4 in]
      n163 = call <vilib>:"DAQmx Start Task.vi"("task/channels in"=w203, "error in"=w205) -> ("task out"=w234:refnum<k21>, "error out"=w236:errorcluster)  [unwired: 12 in]
      n164 = Generate Occurrence() -> (w195:refnum<k4>)
      n165 = Write to Text File(file (use dialog)=w240, text=w241) -> (refnum out=w237:refnum<file>)  [unwired: 2 in, 2 out]
      n166 = call <vilib>:"Obtain Semaphore Reference.vi"("name (unnamed)"="CAN") -> ("semaphore"=w196:T25)  [unwired: 4 in, 2 out]
    }
    frame #3 {
      w274 = u32 0 ("millisecond timer value")
      n167 = call <vilib>:"High Resolution Relative Seconds.vi"() -> ("relative seconds"=w312:dbl)
      n168 = while {
        shift-right: [w863] -> w294
        shift-left: w316 -> [w865]
        tunnel: w314 -> [w872]
        tunnel: w313 -> [w871]
        tunnel: w291 -> [w867]
        shift-right: [w860] -> _
        shift-left: w315 -> [w866]
        tunnel: w292 -> [w856]
        stop <- w857 stop-if-true
        w873 = 2 items=["Zero in progress", "Perform flowmeter zeroing", "Mass flow rate", "Density", "Temperature", "Volume flow rate", "Pressure (internally derived)", "Mass total", "Volume total", "Mass inventory", "Volume inventory", "Start/stop all totalizers", "Reset all totalizers", "Reset all inventories", "Real-time interrupt failure", "Sensor failure", "Temperature sensor failure", "Flowmeter zeroing failure", "Other failure occurred", "Mass flow rate meter factor", "Volume flow rate meter factor", "Density meter factor", "Flowing density calibration constant", "Mass flow scale factor", "Density scale factor", "Temperature scale factor", "Volume flow scale factor", "Pressure scale factor", "Mass total scale factor", "Volume total scale factor", "Mass inventory scale factor", "Volume inventory scale factor", "Flowmeter zeroing standard deviantion (units in microsec)", "Standard or special mass flow unit", "Density unit", "Temperature unit", "Standard or special volume flow unit", "Pressure unit", "Standard or special mass total or inventory unit", "Standard or special volume total or inventory unit", "Base mass unit for special mass unit", "Base time uni for special mass unit", "Base volume unit for special volume unit", "Base time unit for special volume unit", "Maximum zeroing time", "Flow direction", "EEProm checksum failure", "EEProm checksum failure in core processor", "EEProm database corrupt", "RAM diagnostic failure", "RAM diagnostic failure in core processor", "Real-time Interrupt failure", "Watchdog timer error", "Mass flow cutoff", "Volume flow cutoff", "Integer de erro 001", "Slug flow high-density limit (g/cm3)", "Slug flow low-density limit (g/cm3)"] ("Descrição da função leitura")
        # "Leitura do fluxímetro"
        n169 = call <vilib>:"High Resolution Relative Seconds.vi"() -> ("relative seconds"=w870:dbl)
        n170 = feedback #1(w867) -> (w869:dbl)
        n171 = feedback-in #1(w870) -> ()
        n172 = Subtract(x=w870, y=w869) -> (x-y=→"dt - Leitura Fluxímetro [s]":dbl)
        n173 = call "FluxRead.vi"("Error In"=w866, "Função de Leitura"=w873, "Master In"=w865) -> ("Error Out"=w854:errorcluster, "Data"=w862:dbl, "Master Out"=w864:refnum<class "Modbus Master.lvclass">)
        "Erro Fluximetro" <- w854
        n174 = case shown="Error" w854 {
          selector: w854 -> [w875 _]
          tunnel: w864 -> [w876 w879]
          tunnel: [w876 w885] -> w863
          tunnel: [w875 w882] -> w860
          tunnel: w872 -> [_ w884]
          tunnel: w871 -> [_ w883]
          tunnel: w862 -> [w874 w878]
          tunnel: [w874 w877] -> w861
          frame No Error {
          }
          frame Error {
            n175 = flat-sequence {
              tunnel: w883 -> [w887]
              tunnel: w884 -> [w888]
              tunnel: [w888] -> w881
              tunnel: [w887] -> w880
              tunnel: w879 -> [w886]
              tunnel: [w892] -> w885
              tunnel: [w889] -> w882
              tunnel: w881 -> [w891]
              tunnel: w880 -> [w890]
              frame #0 {
                n176 = call "FluxClose.vi"("Master In"=w886) -> ()  [unwired: 1 in, 1 out]
              }
              frame #1 {
                n177 = call "FluxCreate.vi"("Endereço slave"=w891, "Recurso VISA"=w890) -> ("Error Out"=w889:errorcluster, "Master Out"=w892:refnum<class "Modbus Master.lvclass">)
              }
            }
            n178 = feedback-in #2(w878) -> ()
            n179 = feedback #2() -> (w877:dbl)  [unwired: 1 in]
          }
        }
        "Vazão Mássica [kg/h]" <- w861
        n180 = Wait on Occurrence(1:FALSE ("ignore previous (T)"), 2:w856, 3:1000 ("ms timeout (-1)")) -> (0:w859:bool)
        n181 = Not(x=w859) -> (.not. x?=w857:bool)
      }
      n182 = call-poly <vilib>:"DAQmx Write.vi"("task/channels in"=w280, "data"=FALSE) -> ("task out"=w279:refnum<k21>)  [unwired: 11 in, 2 out]
      n183 = call <vilib>:"High Resolution Relative Seconds.vi"() -> ("relative seconds"=w298:dbl)
      n184 = while {
        tunnel: w298 -> [w415]
        tunnel: [w405] -> w324
        tunnel: [w404] -> _
        tunnel: [w398] -> w323
        tunnel: [w397] -> _
        tunnel: [w410] -> _
        tunnel: w307 -> [w412]
        tunnel: w306 -> [w411]
        tunnel: w305 -> [w407]
        tunnel: w304 -> [w406]
        tunnel: w303 -> [w401]
        tunnel: w302 -> [w399]
        tunnel: w301 -> [w392]
        shift-right: [w391] -> w322
        shift-left: w300 -> [w352]
        tunnel: [w345] -> _
        tunnel: w299 -> [w390]
        tunnel: w292 -> [w389]
        tunnel: [w384] -> w293
        tunnel: w290 -> [w376]
        tunnel: w289 -> [w375]
        tunnel: w288 -> [w374]
        tunnel: errorcluster {"status"=FALSE, "code"=0, "source"=""} ("error out") -> [w373]
        tunnel: [w372] -> w285
        tunnel: [w371] -> _
        tunnel: [w370] -> w284
        tunnel: w279 -> [w364]
        tunnel: [w353] -> w277
        shift-right: [w348] -> w262
        shift-left: w266 -> [w349]
        tunnel: w265 -> [_]
        stop <- w386 stop-if-true
        # "Leitura de Pressões (Soma 1 -> Absoluta)"
        # "Leitura Pressão/ Leitura Posição/ Atuação PSuc/ Atuação Temperatura/ Liga e desliga Vent e Comp"
        n185 = flat-sequence {
          tunnel: w364 -> [w460]
          tunnel: [w459] -> w359
          tunnel: [w464] -> w413
          tunnel: w359 -> [w462]
          tunnel: [w462] -> w358
          tunnel: w412 -> [w470]
          tunnel: w411 -> [w469]
          tunnel: [w468] -> w410
          tunnel: [w467] -> w409
          tunnel: [w466] -> w384
          tunnel: w358 -> [w465]
          tunnel: [w465] -> w357
          tunnel: w408 -> [w473]
          tunnel: w357 -> [w471]
          tunnel: [w471] -> w356
          tunnel: w393 -> [w479]
          tunnel: w392 -> [w481]
          tunnel: [w480] -> w391
          tunnel: w356 -> [w478]
          tunnel: [w478] -> w351
          tunnel: w352 -> [w477]
          tunnel: w337 -> [w476]
          tunnel: "Frequência PWM [Hz]" -> [w475]
          tunnel: [w474] -> w346
          tunnel: w351 -> [w497]
          tunnel: [w497] -> w350
          tunnel: [w496] -> w348
          tunnel: [w495] -> w345
          tunnel: w333 -> [w494]
          tunnel: "Frequência PWM [Hz]" -> [w493]
          tunnel: w349 -> [w492]
          tunnel: w346 -> [w491]
          tunnel: w341 -> [w490]
          tunnel: w407 -> [w511]
          tunnel: w406 -> [w510]
          tunnel: [w509] -> w403
          tunnel: [w508] -> w402
          tunnel: w383 -> [w506]
          tunnel: w350 -> [w507]
          tunnel: [w507] -> w355
          tunnel: w403 -> [w519]
          tunnel: w402 -> [w518]
          tunnel: w401 -> [w517]
          tunnel: w400 -> [w512]
          tunnel: w399 -> [w516]
          tunnel: [w519] -> w363
          tunnel: [w518] -> w362
          tunnel: [w515] -> w361
          tunnel: [w514] -> w360
          tunnel: w355 -> [w513]
          tunnel: [w513] -> w354
          tunnel: [w523] -> w397
          tunnel: [w524] -> w398
          tunnel: [w525] -> w404
          tunnel: [w526] -> w405
          tunnel: w363 -> [w526]
          tunnel: w362 -> [w525]
          tunnel: w361 -> [w524]
          tunnel: w360 -> [w523]
          tunnel: w354 -> [w521]
          tunnel: [w520] -> w353
          frame #0 {
            # "Timer pulse up"
            n186 = call-poly <vilib>:"DAQmx Write.vi"("task/channels in"=w460, "data"=TRUE) -> ("task out"=w459:refnum<k21>)  [unwired: 11 in, 2 out]
          }
          frame #1 {
            # "Pressão"
            n187 = call "DAQ Assistant"() -> ("data"=w464:dynamicdata, "error out"=→"Erro Pressão":errorcluster)  [unwired: 17 in, 1 out]
          }
          frame #2 {
            # "Encoder"
            n188 = call "Encoder Read.vi"("error in (no error)"=w470, "Task In"=w469) -> ("error out"=w468:errorcluster, "Posição"=w467:i32, "Task Out"=w466:T24)  [unwired: 7 in]
          }
          frame #3 {
            # "Valv. Sucção"
            n189 = call "DAQ Assistant2"("data"=w473) -> ("error out"=→"Erro Valv. Sucção":errorcluster)  [unwired: 17 in, 1 out]
          }
          frame #4 {
            # "Resistência Descarga"
            n190 = case shown="True" w479 {
              tunnel: w475 -> [_ w489]
              tunnel: w476 -> [_ w488]
              tunnel: w477 -> [w483 w487]
              tunnel: w481 -> [w482 w486]
              tunnel: [w483 w485] -> w480
              tunnel: [w482 w484] -> w474
              frame False {
              }
              frame True {
                n191 = call-poly <vilib>:"DAQmx Write.vi"("task/channels in"=w487, "frequency"=w489, "duty cycle"=w488, "error in"=w486) -> ("task out"=w485:refnum<k21>, "error out"=w484:errorcluster)  [unwired: 9 in, 1 out]
              }
            }
          }
          frame #5 {
            # "Resistência Sucção"
            n192 = case shown="True" w490 {
              tunnel: w493 -> [_ w505]
              tunnel: w494 -> [_ w504]
              tunnel: w492 -> [w499 w503]
              tunnel: w491 -> [w498 w502]
              tunnel: [w499 w501] -> w496
              tunnel: [w498 w500] -> w495
              frame False {
              }
              frame True {
                n193 = call-poly <vilib>:"DAQmx Write.vi"("task/channels in"=w503, "frequency"=w505, "duty cycle"=w504, "error in"=w502) -> ("task out"=w501:refnum<k21>, "error out"=w500:errorcluster)  [unwired: 9 in, 1 out]
              }
            }
          }
          frame #6 {
            # "Vnetilador"
            n194 = call-poly <vilib>:"DAQmx Write.vi"("task/channels in"=w511, "data"=w506, "error in"=w510) -> ("task out"=w509:refnum<k21>, "error out"=w508:errorcluster)  [unwired: 10 in, 1 out]
          }
          frame #7 {
            # "Compressor"
            n195 = call-poly <vilib>:"DAQmx Write.vi"("task/channels in"=w517, "data"=w512, "error in"=w516) -> ("task out"=w515:refnum<k21>, "error out"=w514:errorcluster)  [unwired: 10 in, 1 out]
          }
          frame #8 {
            # "Timer pulse down"
            n196 = call-poly <vilib>:"DAQmx Write.vi"("task/channels in"=w521, "data"=FALSE) -> ("task out"=w520:refnum<k21>)  [unwired: 11 in, 2 out]
          }
        }
        n197 = call <vilib>:"High Resolution Relative Seconds.vi"() -> ("relative seconds"=w427:dbl)
        n198 = Split Signals(w413) -> (w429:dynamicdata, w430:dynamicdata, w433:dynamicdata)  [unwired: 3 in]
        n199 = feedback #3(w415) -> (w428:dbl)
        n200 = Subtract(x=w427, y=w428) -> (x-y=→"dt - At PressãoTemp/Le Pos":dbl)
        n201 = feedback-in #3(w427) -> ()
        n202 = Wait on Occurrence(1:FALSE ("ignore previous (T)"), 2:w389, 3:320 ("ms timeout (-1)")) -> (0:w388:bool)
        n203 = call "Convert from Dynamic Data2"("Dynamic Data Type"=w429) -> ("Array"=w424:dbl[])  [unwired: 3 in]
        n204 = call "Convert from Dynamic Data"("Dynamic Data Type"=w430) -> ("Array"=w425:dbl[])  [unwired: 3 in]
        n205 = call "Convert from Dynamic Data9"("Dynamic Data Type"=w433) -> ("Array"=w434:dbl[])  [unwired: 3 in]
        n206 = Not(x=w388) -> (.not. x?=w386:bool)
        n207 = local read "Tensão da válvula de sucção [V]"() -> (w408:dbl)
        n208 = call <vilib>:"Std Deviation and Variance.vi"("X"=w434) -> ("mean"=w435:dbl)  [unwired: 1 in, 2 out]
        n209 = call <vilib>:"Std Deviation and Variance.vi"("X"=w425) -> ("mean"=w419:dbl)  [unwired: 1 in, 2 out]
        n210 = call <vilib>:"Std Deviation and Variance.vi"("X"=w424) -> ("mean"=w417:dbl)  [unwired: 1 in, 2 out]
        n211 = flat-sequence {
          tunnel: w376 -> [w439]
          tunnel: w375 -> [w442]
          tunnel: [w442] -> w382
          tunnel: [w439] -> w381
          tunnel: [w441] -> w380
          tunnel: w374 -> [w440]
          tunnel: [w448] -> w379
          tunnel: [w447] -> w378
          tunnel: w382 -> [w449]
          tunnel: w381 -> [w443]
          tunnel: w380 -> [w446]
          tunnel: [w446] -> w377
          tunnel: w373 -> [w445]
          tunnel: [w444] -> w371
          tunnel: [w443] -> w370
          tunnel: [w457] -> w372
          tunnel: [w458] -> w366
          tunnel: w379 -> [w458]
          tunnel: w378 -> [w457]
          tunnel: w377 -> [w456]
          frame #0 {
            n212 = call <vilib>:"Acquire Semaphore.vi"("semaphore"=w440) -> ("semaphore out"=w441:T25)  [unwired: 4 in, 2 out]
          }
          frame #1 {
            n213 = for {
              tunnel: [w454] -> w448 mode=indexing
              shift-right: [w451] -> w444
              shift-left: w445 -> [w452]
              shift-right: [w453] -> w447
              shift-left: w449 -> [w455]
              tunnel: w443 -> [w450] mode=indexing
              n214 = call "GPSPressCANRead.vi"("Error In"=w452, "NodeID"=w450, "ObjHandle In"=w455) -> ("Error Out"=w451:errorcluster, "Pressure"=w454:sgl, "ObjHandle Out"=w453:u32)  [unwired: 6 in]
            }
          }
          frame #2 {
            n215 = call <vilib>:"Release Semaphore.vi"("semaphore"=w456) -> ()  [unwired: 5 in, 2 out]
          }
        }
        n216 = local read "Duty Cycle da Resistência [%]"() -> (w330:dbl)
        n217 = local read "Duty Cycle da Resistência [%] 2"() -> (w329:dbl)
        n218 = Multiply(x=w435, y=6.0) -> (x*y=w436:dbl)
        n219 = Multiply(x=w419, y=6.0) -> (x*y=w422:dbl)
        n220 = Multiply(x=w417, y=6.0) -> (x*y=w423:dbl)
        n221 = Add(x=w436, y=1.0) -> (x+y=→"Intermed [bar]":dbl)
        n222 = Add(x=w423, y=1.0) -> (x+y=→"Sucção [bar]":dbl)
        n223 = Add(x=w422, y=1.0) -> (x+y=→"Descarga [bar]":dbl)
        n224 = Divide(x=w330, y=100.0) -> (x/y=w336:dbl)
        n225 = Divide(x=w329, y=100.0) -> (x/y=w331:dbl)
        n226 = feedback #4(w390) -> (w396:dbl)
        n227 = feedback-in #4("Frequência PWM [Hz]") -> ()
        n228 = Index Array(array=w366, index #1=0 ("index"), index #2=1 ("index")) -> (element #1=→"GE Valv S [bar]":sgl, element #2=→"GE Comp S [bar]":sgl)
        n229 = In Range and Coerce(upper limit=0.99999988 ("output high"), x=w336, lower limit=1.19209297e-07 ("output low")) -> (coerced(x)=w337:dbl)  [unwired: 1 out]
        n230 = In Range and Coerce(upper limit=0.99999988 ("output high"), x=w331, lower limit=1.19209297e-07 ("output low")) -> (coerced(x)=w333:dbl)  [unwired: 1 out]
        n231 = feedback #5() -> (w395:dbl)  [unwired: 1 in]
        n232 = feedback-in #5(w337) -> ()
        n233 = feedback #6() -> (w344:dbl)  [unwired: 1 in]
        n234 = feedback-in #6(w333) -> ()
        n235 = Not Equal?(x="Frequência PWM [Hz]", y=w396) -> (x != y?=w343:bool)
        n236 = case shown="False" w386 {
          tunnel: ["Ativar Compressor?" w529] -> w400
          tunnel: ["Ativar Ventilador?" w529] -> w383
          frame False {
            # "Pode iniciar"
          }
          frame True {
            w529 = FALSE
            # "Stop"
            n237 = local write "Ativar Compressor?"(w529) -> ()
          }
        }
        n238 = Not Equal?(x=w333, y=w344) -> (x != y?=w342:bool)
        n239 = Not Equal?(x=w337, y=w395) -> (x != y?=w394:bool)
        n240 = Or(x=w343, y=w394) -> (x .or. y?=w393:bool)
        n241 = Or(x=w342, y=w343) -> (x .or. y?=w341:bool)
        "Posição Atual da Válvula de Descarga" <- w409
      }
      n242 = while {
        tunnel: w312 -> [w811]
        shift-right: [w844] -> _
        shift-left: w311 -> [w847]
        tunnel: w310 -> [w838]
        tunnel: w308 -> [w815]
        tunnel: w292 -> [w803]
        tunnel: [w793] -> _
        tunnel: w273 -> [w793]
        tunnel: w272 -> [w791]
        tunnel: [w787] -> w271
        tunnel: [w786] -> w270
        tunnel: w269 -> [w770]
        i -> [w772]
        stop <- w802 stop-if-true
        w788 = u16 2  # Power
        w789 = u16 0  # Voltage
        w795 = u16 1  # Current
        # "Lê Vibrações"
        # "Lê Corrente Compressor"
        # "Lê Emissõoes Acústicas"
        # "Le corrente e vib/Salva as medições"
        n243 = call <vilib>:"High Resolution Relative Seconds.vi"() -> ("relative seconds"=w810:dbl)
        n244 = feedback #7(w811) -> (w849:dbl)
        n245 = feedback-in #7(w810) -> ()
        n246 = flat-sequence {
          tunnel: [w852] -> w754
          tunnel: [w851] -> w765
          tunnel: [w850] -> w759
          frame #0 {
            n247 = global read "FPGA_RW_Vars.vi" "Vibration (NI-9234)"() -> (w850:T26)
            n248 = global read "FPGA_RW_Vars.vi" "Voltage (NI-9225)"() -> (w853:cluster{"Voltage (CH0)":waveform(dbl)})
            n249 = global read "FPGA_RW_Vars.vi" "Voltage (NI-9215)"() -> (w851:T27)
            n250 = Unbundle By Name(w853) -> ("Voltage (CH0)"=w852:waveform(dbl))
          }
        }
        n251 = Wait on Occurrence(1:FALSE ("ignore previous (T)"), 2:w803, 3:60000 ("ms timeout (-1)")) -> (0:w805:bool)
        n252 = Subtract(x=w810, y=w849) -> (x-y=→"dt - Salvar dados [s]":dbl)
        n253 = Subtract(x=w810, y=w811) -> (x-y=w809:dbl)
        n254 = Quotient & Remainder(x=w772, y=10) -> (x-y*floor(x/y)=w806:i32)  [unwired: 1 out]
        n255 = Not(x=w805) -> (.not. x?=w802:bool)
        n256 = Equal To 0?(x=w806) -> ()  [unwired: 1 out]
        n257 = Number To Decimal String(number=w772) -> (decimal integer string=w840:string)  [unwired: 1 in]
        n258 = Number To Decimal String(number=w772) -> (decimal integer string=w774:string)  [unwired: 1 in]
        n259 = Number To Decimal String(number=w772) -> (decimal integer string=w818:string)  [unwired: 1 in]
        n260 = Unbundle By Name(w759) -> ("Vibration Lower (CH0)"=w758:waveform(dbl), "Vibration Dummy (CH1)"=w757:waveform(dbl), "Vibration Upper (CH2)"=w756:waveform(dbl))
        n261 = call <instrlib>:"Read Normal Measurement.vi"("error in (no error)"=w791, "Item (0: V)"=w789, "VISA resource name"=w793) -> ("error out"=w784:errorcluster, "Value"=w783:dbl, "VISA resource name out"=w792:refnum<visa-resource-name>)  [unwired: 5 in, 1 out]
        "Tensão RMS [V] (WT130)" <- w783
        n262 = Concatenate Strings("Nome de Base do Arquivo - Vibração", w840, ".dat" ("string")) -> (w839:string)
        n263 = Concatenate Strings("Nome de Base do Arquivo - Tensão", w774, ".dat" ("string")) -> (w775:string)
        n264 = Concatenate Strings("Nome de Base do Arquivo - Corrente", w818, ".dat" ("string")) -> (w817:string)
        n265 = call <instrlib>:"Read Normal Measurement.vi"("error in (no error)"=w784, "Item (0: V)"=w795, "VISA resource name"=w792) -> ("error out"=w785:errorcluster, "Value"=w794:dbl, "VISA resource name out"=w790:refnum<visa-resource-name>)  [unwired: 5 in, 1 out]
        "Corrente RMS [A] (WT130)" <- w794
        n266 = Unbundle By Name(w765) -> ("Voltage LEM (CH0)"=w764:waveform(dbl), "Voltage TMCS (CH2)"=w763:waveform(dbl))
        n267 = Build Path(base path=w838, name or relative path=w839) -> (appended path=w812:path)
        n268 = Build Path(base path=w770, name or relative path=w775) -> (appended path=w771:path)
        n269 = Build Path(base path=w815, name or relative path=w817) -> (appended path=w813:path)
        n270 = Build Array(w758, w757, w756) -> (w755:waveform(dbl)[])
        n271 = call <instrlib>:"Read Normal Measurement.vi"("error in (no error)"=w785, "Item (0: V)"=w788, "VISA resource name"=w790) -> ("error out"=w786:errorcluster, "Value"=w782:dbl, "VISA resource name out"=w787:refnum<visa-resource-name>)  [unwired: 5 in, 1 out]
        "Potência [W] (WT130)" <- w782
        n272 = local read "Corrente RMS [A] (LEM)"() -> (w826:dbl)
        n273 = local read "Tensão da válvula de sucção [V]"() -> (w799:dbl)
        n274 = local read "Ativar Compressor?"() -> (w832:bool)
        n275 = local read "Setpoint da abertura da valvula"() -> (w827:dbl)
        n276 = local read "Posição Atual da Válvula de Descarga"() -> (w830:dbl)
        n277 = local read "Limite inferior da posição da válvula"() -> (w800:dbl)
        n278 = call-poly <vilib>:"Write Waveforms to File.vi"("waveform array"=w755, "file path (dialog if empty)"=w812) -> ()  [unwired: 8 in, 2 out]
        n279 = Multiply(x=w764, y=10.0) -> (x*y=w760:waveform(dbl))
        n280 = call-poly <vilib>:"Write Waveforms to File.vi"("waveform"=w754, "file path (dialog if empty)"=w771) -> ()  [unwired: 8 in, 2 out]
        n281 = Reciprocal(x=0.4 ("y")) -> (1/x=w781:dbl)
        n282 = call-poly <vilib>:"RMS.vi"("X"=w758) -> ("rms value"=w835:dbl)  [unwired: 1 out]
        "RMS Inferior [g]" <- w835
        n283 = call-poly <vilib>:"RMS.vi"("X"=w757) -> ("rms value"=w836:dbl)  [unwired: 1 out]
        "RMS Bancada [g]" <- w836
        n284 = call-poly <vilib>:"RMS.vi"("X"=w756) -> ("rms value"=w834:dbl)  [unwired: 1 out]
        "RMS Superior [g]" <- w834
        n285 = Multiply(x=w781, y=w763) -> (x*y=w762:waveform(dbl))
        n286 = call-poly <vilib>:"RMS.vi"("X"=w760) -> ("rms value"=→"Corrente RMS [A] (LEM)":dbl)  [unwired: 1 out]
        n287 = Build Array(w760, w762) -> (w761:waveform(dbl)[])
        n288 = local read "Corrente RMS [A] (TMCS)"() -> (w779:dbl)
        n289 = local read "Bobina 1 [ºC]"() -> (w777:dbl)
        n290 = local read "Bobina 2 [ºC]"() -> (w821:dbl)
        n291 = local read "Descarga [bar]"() -> (w825:dbl)
        n292 = local read "Descarga [ºC]"() -> (w823:dbl)
        n293 = local read "Sucção [bar]"() -> (w824:dbl)
        n294 = local read "Intermed [bar]"() -> (w808:dbl)
        n295 = Build Array(w835, w836, w834) -> (w842:dbl[])
        "Acc" <- w842
        n296 = local read "Sucção [ºC]"() -> (w822:dbl)
        n297 = call-poly <vilib>:"Write Waveforms to File.vi"("waveform array"=w761, "file path (dialog if empty)"=w813) -> ()  [unwired: 8 in, 2 out]
        n298 = call-poly <vilib>:"RMS.vi"("X"=w762) -> ("rms value"=→"Corrente RMS [A] (TMCS)":dbl)  [unwired: 1 out]
        n299 = call-poly <vilib>:"RMS.vi"("X"=w754) -> ("rms value"=w769:dbl)  [unwired: 1 out]
        "Tensão RMS [V] (DAQ)" <- w769
        n300 = Subtract(x=w830, y=w800) -> (x-y=w829:dbl)
        n301 = Subtract(x=w827, y=w800) -> (x-y=w828:dbl)
        n302 = local read "Reservatório [ºC]"() -> (w766:dbl)
        n303 = local read "Ambiente [ºC]"() -> (w767:dbl)
        n304 = Boolean To (0,1)(Boolean=w832) -> (0, 1=w831:i16)
        n305 = local read "Corpo [ºC]"() -> (w768:dbl)
        n306 = local read "GE Comp S [bar]"() -> (w796:dbl)
        n307 = local read "GE Valv S [bar]"() -> (w797:dbl)
        n308 = local read "Vazão Mássica [kg/h]"() -> (w833:dbl)
        n309 = local read "Duty Cycle da Resistência [%]"() -> (w798:dbl)
        n310 = Build Array (concatenate)(w809, w777, w821, w822, w823, w824, w825, w808, w828, w829, w800, w799, w826, w831, w842, w833, w798, w797, w796, w794, w783, w782, w779, w769, w768, w767, w766) -> (w843:dbl[])
        n311 = Array To Spreadsheet String(array=w843, 3:"%#_10g" ("text")) -> (spreadsheet string=w845:string)  [unwired: 1 in]
        n312 = Write to Text File(file (use dialog)=w847, text=w845) -> (refnum out=w844:refnum<file>)  [unwired: 2 in, 2 out]
      }
      n313 = call <vilib>:"High Resolution Relative Seconds.vi"() -> ("relative seconds"=w309:dbl)
      n314 = call "FluxClose.vi"("Master In"=w294) -> ()  [unwired: 1 in, 1 out]
      n315 = while {
        tunnel: w309 -> [w730]
        tunnel: w292 -> [w729]
        stop <- w739 stop-if-true
        # "Controle da resistência"
        # "Leitura e Controle de Temperatura"
        n316 = global read "FPGA_RW_Vars.vi" "Temperature 2 (NI-9219)"() -> (w710:T28)
        n317 = global read "FPGA_RW_Vars.vi" "Temperature (NI-9219)"() -> (w715:T28)
        n318 = call <vilib>:"High Resolution Relative Seconds.vi"() -> ("relative seconds"=w731:dbl)
        n319 = Wait on Occurrence(1:FALSE ("ignore previous (T)"), 2:w729, 3:1000 ("ms timeout (-1)")) -> (0:w741:bool)
        n320 = Not(x=w741) -> (.not. x?=w739:bool)
        n321 = feedback #8(w730) -> (w753:dbl)
        n322 = Subtract(x=w731, y=w753) -> (x-y=→"dt - Leitura Temperatura [s]":dbl)
        n323 = feedback-in #8(w731) -> ()
        n324 = Unbundle By Name(w715) -> ("Temperature (CH0)"=→"Bobina 1 [ºC]":dbl, "Temperature (CH1)"=→"Bobina 2 [ºC]":dbl, "Temperature (CH2)"=w714:dbl, "Temperature (CH3)"=w713:dbl)
        "Sucção [ºC]" <- w714
        "Descarga [ºC]" <- w713
        n325 = Unbundle By Name(w710) -> ("Temperature (CH0)"=→"Corpo [ºC]":dbl, "Temperature (CH1)"=→"Ambiente [ºC]":dbl, "Temperature (CH2)"=→"Reservatório [ºC]":dbl)
        n326 = Divide(x="Limite Superior DC Auto [%]", y=100.0) -> (x/y=w734:dbl)
        n327 = Bundle(w734, "output low"=1.19209297e-07) -> (w727:cluster{dbl, "output low":dbl})  [unwired: 1 in]
        n328 = Divide(x="DC da Resistência (Des) [%]", y=100.0) -> (x/y=w732:dbl)
        n329 = call-poly <vilib>:"PID Advanced.vi"("setpoint"="Setpoint T. Desc. [ºC]", "output range"=w727, "auto? (T)"="Temp. Desc. Auto?", "manual control"=w732, "process variable"=w713, "PID gains"="Ganhos - Temperatura Descarga") -> ("output"=w747:dbl)  [unwired: 8 in, 1 out]
        n330 = Divide(x="DC da Resistência (Suc) [%]", y=100.0) -> (x/y=w717:dbl)
        n331 = In Range and Coerce(upper limit=0.999999881 ("output high"), x=w717, lower limit=1.19209297e-07 ("output low")) -> (coerced(x)=w718:dbl)  [unwired: 1 out]
        n332 = In Range and Coerce(upper limit=0.999999881 ("output high"), x=w747, lower limit=1.19209297e-07 ("output low")) -> (coerced(x)=w746:dbl)  [unwired: 1 out]
        n333 = call "Convert from Dynamic Data14"("Dynamic Data Type"=w714) -> ("Scalar"=w725:dbl)  [unwired: 3 in]
        n334 = Multiply(x=w718, y=100.0) -> (x*y=→"Duty Cycle da Resistência [%] 2":dbl)
        n335 = Multiply(x=w746, y=100.0) -> (x*y=→"Duty Cycle da Resistência [%]":dbl)
        n336 = call-poly <vilib>:"PID Advanced.vi"("setpoint"="Setpoint T. Suc. [ºC]", "output range"=w727, "auto? (T)"="Temp. Suc. Auto?", "manual control"=w717, "process variable"=w725, "PID gains"="Ganhos - Temperatura Sucção") -> ()  [unwired: 8 in, 2 out]
        "T.D. Auto?" <- "Temp. Desc. Auto?"
        "T.S. Auto?" <- "Temp. Suc. Auto?"
      }
      n337 = call <vilib>:"High Resolution Relative Seconds.vi"() -> ("relative seconds"=w297:dbl)
      n338 = while {
        tunnel: w297 -> [w588]
        tunnel: w292 -> [w563]
        shift-right: [w545] -> _
        shift-left: FALSE -> [w550]
        shift-right: [w544] -> _
        shift-left: w274 -> [w547]
        shift-right: [w543] -> _
        shift-left: w274 -> [w546]
        stop <- w562 stop-if-true
        # "Erros de Atuação"
        # "Erros de Leitura"
        # "Limpa Gráficos"
        # "Atualiza Gráficos"
        n339 = local read "Corrente RMS [A] (WT130)"() -> (w539:dbl)
        n340 = local read "Corrente RMS [A] (LEM)"() -> (w541:dbl)
        n341 = disable-structure shown="Disabled" {
          frame Disabled {
            n342 = local read "Duty Cycle da Resistência [%]"() -> (→"DC":dbl)
          }
          frame Enabled {
          }
        }
        n343 = local read "GE Valv S [bar]"() -> (w555:dbl)
        n344 = local read "GE Comp S [bar]"() -> (w552:dbl)
        n345 = local read "Intermed [bar]"() -> (w566:dbl)
        n346 = local read "Setpoint Descarga [bar]"() -> (w572:dbl)
        n347 = local read "Vazão Mássica [kg/h]"() -> (→"Grafico Vazão" →"G Vazão":dbl)
        n348 = local read "Setpoint Sucção [bar]"() -> (w573:dbl)
        n349 = local read "Descarga [bar]"() -> (w571:dbl)
        n350 = local read "Sucção [bar]"() -> (w554:dbl)
        n351 = local read "Intermed [bar]"() -> (→"G Pressão Intermed":dbl)
        n352 = feedback #9(w588) -> (w590:dbl)
        n353 = call <vilib>:"High Resolution Relative Seconds.vi"() -> ("relative seconds"=w591:dbl)
        n354 = feedback-in #9(w591) -> ()
        n355 = disable-structure shown="Enabled" {
          disable-tunnel: w554 -> [w619 _]
          disable-tunnel: [w619 w620] -> w553
          disable-tunnel: w552 -> [_ w620]
          frame Disabled {
          }
          frame Enabled {
          }
        }
        n356 = Subtract(x=w591, y=w590) -> (x-y=→"dt - Atualiza Gráficos [s]":dbl)
        n357 = Bundle("Corrente RMS [A] (LEM)"=w541, "Corrente RMS [A] (WT130)"=w539) -> (→"Grafico Corrente" →"G Corrente RMS":T29)  [unwired: 1 in]
        n358 = Bundle("Sucção [bar]"=w554, "Descarga [bar]"=w571, "Intermed [bar]"=w566, "GE Valv S [bar]"=w555, "GE Comp S [bar]"=w552) -> (→"Grafico Pressão":T3)  [unwired: 1 in]
        n359 = Bundle("Descarga [bar]"=w571, "Setpoint Descarga [bar]"=w572) -> (→"G Pressão de Descarga":T30)  [unwired: 1 in]
        n360 = Bundle("GE Comp S [bar]"=w553, "Setpoint Sucção [bar]"=w573) -> (→"G Pressão de Sucção":T31)  [unwired: 1 in]
        n361 = local read "Ativar Compressor?"() -> (w551:bool)
        n362 = Build Array(w551, w550) -> (w549:bool[])
        n363 = local read "Abertura Atual da Válvula de Descarga"() -> (w570:dbl)
        n364 = local read "Tensão da válvula de sucção [V]"() -> (→"G Tensão na válvula de Sucção":dbl)
        n365 = local read "Velocidade do motor de descarga"() -> (→"G Vel. do Motor da Válvula de Descarga":dbl)
        n366 = local read "Setpoint da abertura da valvula"() -> (w569:dbl)
        n367 = Boolean Array To Number(Boolean array=w549) -> (number=w548:u32)
        n368 = case shown="1" w548 {
          tunnel: w547 -> [w606 _ w613 w616]
          tunnel: w546 -> [w607 w609 w614 _]
          tunnel: [w607 w609 w614 w617] -> w543
          tunnel: [FALSE TRUE FALSE TRUE] -> w545
          tunnel: [w606 w611 w613 w616] -> w544
          frame 0, Default {
          }
          frame 1 {
            n369 = Tick Count (ms)() -> (millisecond timer value=w611:u32)
          }
          frame 2 {
          }
          frame 3 {
            n370 = Tick Count (ms)() -> (millisecond timer value=w618:u32)
            n371 = Subtract(x=w618, y=w616) -> (x-y=w617:u32)
          }
        }
        n372 = event shown="[1] \"Eixo X\": Value Change" {
          selector: _ -> [_ _ _]
          dyn-events: _ -> [_ _ _]
          timeout: 500 -> [_ _ _]
          event Timeout {
            n373 = event-data() -> ()  [unwired: 1 in, 3 out]
          }
          event "Eixo X": Value Change {
            n374 = event-data() -> ("NewVal"=w592:u16)  [unwired: 1 in, 5 out]
            n375 = case shown="3" w592 {
              frame 0, Default {
                w594 = "Amostras" ("X Scale.Name Label.Text")
                w593 = 1.0 ("X Scale.Offset and Multiplier:Multiplier")
                n376 = property on="G Corrente RMS" class="WFChart (strict)"("XScale.Multiplier"=w593, "XScale.NameLbl.Text"=w594) -> ()  [unwired: 2 in, 2 out]
                n377 = property on="G Posição do Encoder" class="WFChart (strict)"("XScale.Multiplier"=w593, "XScale.NameLbl.Text"=w594) -> ()  [unwired: 2 in, 2 out]
                n378 = property on="G Pressão Intermed" class="WFChart (strict)"("XScale.Multiplier"=w593, "XScale.NameLbl.Text"=w594) -> ()  [unwired: 2 in, 2 out]
                n379 = property on="G Pressão de Descarga" class="WFChart (strict)"("XScale.Multiplier"=w593, "XScale.NameLbl.Text"=w594) -> ()  [unwired: 2 in, 2 out]
                n380 = property on="G Pressão de Sucção" class="WFChart (strict)"("XScale.Multiplier"=w593, "XScale.NameLbl.Text"=w594) -> ()  [unwired: 2 in, 2 out]
                n381 = property on="G Temperaturas" class="WFChart (strict)"("XScale.Multiplier"=w593, "XScale.NameLbl.Text"=w594) -> ()  [unwired: 2 in, 2 out]
                n382 = property on="G Tensão Yokogawa" class="WFChart (strict)"("XScale.Multiplier"=w593, "XScale.NameLbl.Text"=w594) -> ()  [unwired: 2 in, 2 out]
                n383 = property on="G Tensão na válvula de Sucção" class="WFChart (strict)"("XScale.Multiplier"=w593, "XScale.NameLbl.Text"=w594) -> ()  [unwired: 2 in, 2 out]
                n384 = property on="G Vazão" class="WFChart (strict)"("XScale.Multiplier"=w593, "XScale.NameLbl.Text"=w594) -> ()  [unwired: 2 in, 2 out]
                n385 = property on="G Vel. do Motor da Válvula de Descarga" class="WFChart (strict)"("XScale.Multiplier"=w593, "XScale.NameLbl.Text"=w594) -> ()  [unwired: 2 in, 2 out]
                n386 = property on="Grafico Corrente" class="WFChart (strict)"("XScale.Multiplier"=w593, "XScale.NameLbl.Text"=w594) -> ()  [unwired: 2 in, 2 out]
                n387 = property on="Grafico Pressão" class="WFChart (strict)"("XScale.Multiplier"=w593, "XScale.NameLbl.Text"=w594) -> ()  [unwired: 2 in, 2 out]
                n388 = property on="Grafico Temperatura" class="WFChart (strict)"("XScale.Multiplier"=w593, "XScale.NameLbl.Text"=w594) -> ()  [unwired: 2 in, 2 out]
                n389 = property on="Grafico Vazão" class="WFChart (strict)"("XScale.Multiplier"=w593, "XScale.NameLbl.Text"=w594) -> ()  [unwired: 2 in, 2 out]
                n390 = property on="Grafico Vibração" class="WFChart (strict)"("XScale.Multiplier"=w593, "XScale.NameLbl.Text"=w594) -> ()  [unwired: 2 in, 2 out]
              }
              frame 1 {
                w596 = "Tempo [s]" ("X Scale.Name Label.Text")
                w595 = 0.5 ("X Scale.Offset and Multiplier:Multiplier")
                n391 = property on="G Corrente RMS" class="WFChart (strict)"("XScale.Multiplier"=w595, "XScale.NameLbl.Text"=w596) -> ()  [unwired: 2 in, 2 out]
                n392 = property on="G Posição do Encoder" class="WFChart (strict)"("XScale.Multiplier"=w595, "XScale.NameLbl.Text"=w596) -> ()  [unwired: 2 in, 2 out]
                n393 = property on="G Pressão Intermed" class="WFChart (strict)"("XScale.Multiplier"=w595, "XScale.NameLbl.Text"=w596) -> ()  [unwired: 2 in, 2 out]
                n394 = property on="G Pressão de Descarga" class="WFChart (strict)"("XScale.Multiplier"=w595, "XScale.NameLbl.Text"=w596) -> ()  [unwired: 2 in, 2 out]
                n395 = property on="G Pressão de Sucção" class="WFChart (strict)"("XScale.Multiplier"=w595, "XScale.NameLbl.Text"=w596) -> ()  [unwired: 2 in, 2 out]
                n396 = property on="G Temperaturas" class="WFChart (strict)"("XScale.Multiplier"=w595, "XScale.NameLbl.Text"=w596) -> ()  [unwired: 2 in, 2 out]
                n397 = property on="G Tensão Yokogawa" class="WFChart (strict)"("XScale.Multiplier"=w595, "XScale.NameLbl.Text"=w596) -> ()  [unwired: 2 in, 2 out]
                n398 = property on="G Tensão na válvula de Sucção" class="WFChart (strict)"("XScale.Multiplier"=w595, "XScale.NameLbl.Text"=w596) -> ()  [unwired: 2 in, 2 out]
                n399 = property on="G Vazão" class="WFChart (strict)"("XScale.Multiplier"=w595, "XScale.NameLbl.Text"=w596) -> ()  [unwired: 2 in, 2 out]
                n400 = property on="G Vel. do Motor da Válvula de Descarga" class="WFChart (strict)"("XScale.Multiplier"=w595, "XScale.NameLbl.Text"=w596) -> ()  [unwired: 2 in, 2 out]
                n401 = property on="Grafico Corrente" class="WFChart (strict)"("XScale.Multiplier"=w595, "XScale.NameLbl.Text"=w596) -> ()  [unwired: 2 in, 2 out]
                n402 = property on="Grafico Pressão" class="WFChart (strict)"("XScale.Multiplier"=w595, "XScale.NameLbl.Text"=w596) -> ()  [unwired: 2 in, 2 out]
                n403 = property on="Grafico Temperatura" class="WFChart (strict)"("XScale.Multiplier"=w595, "XScale.NameLbl.Text"=w596) -> ()  [unwired: 2 in, 2 out]
                n404 = property on="Grafico Vazão" class="WFChart (strict)"("XScale.Multiplier"=w595, "XScale.NameLbl.Text"=w596) -> ()  [unwired: 2 in, 2 out]
                n405 = property on="Grafico Vibração" class="WFChart (strict)"("XScale.Multiplier"=w595, "XScale.NameLbl.Text"=w596) -> ()  [unwired: 2 in, 2 out]
              }
              frame 2 {
                w600 = "Tempo [min]" ("X Scale.Name Label.Text")
                n406 = Divide(x=0.5 ("X Scale.Offset and Multiplier:Multiplier"), y=60.0) -> (x/y=w597:dbl)
                n407 = property on="G Corrente RMS" class="WFChart (strict)"("XScale.Multiplier"=w597, "XScale.NameLbl.Text"=w600) -> ()  [unwired: 2 in, 2 out]
                n408 = property on="G Posição do Encoder" class="WFChart (strict)"("XScale.Multiplier"=w597, "XScale.NameLbl.Text"=w600) -> ()  [unwired: 2 in, 2 out]
                n409 = property on="G Pressão Intermed" class="WFChart (strict)"("XScale.Multiplier"=w597, "XScale.NameLbl.Text"=w600) -> ()  [unwired: 2 in, 2 out]
                n410 = property on="G Pressão de Descarga" class="WFChart (strict)"("XScale.Multiplier"=w597, "XScale.NameLbl.Text"=w600) -> ()  [unwired: 2 in, 2 out]
                n411 = property on="G Pressão de Sucção" class="WFChart (strict)"("XScale.Multiplier"=w597, "XScale.NameLbl.Text"=w600) -> ()  [unwired: 2 in, 2 out]
                n412 = property on="G Temperaturas" class="WFChart (strict)"("XScale.Multiplier"=w597, "XScale.NameLbl.Text"=w600) -> ()  [unwired: 2 in, 2 out]
                n413 = property on="G Tensão Yokogawa" class="WFChart (strict)"("XScale.Multiplier"=w597, "XScale.NameLbl.Text"=w600) -> ()  [unwired: 2 in, 2 out]
                n414 = property on="G Tensão na válvula de Sucção" class="WFChart (strict)"("XScale.Multiplier"=w597, "XScale.NameLbl.Text"=w600) -> ()  [unwired: 2 in, 2 out]
                n415 = property on="G Vazão" class="WFChart (strict)"("XScale.Multiplier"=w597, "XScale.NameLbl.Text"=w600) -> ()  [unwired: 2 in, 2 out]
                n416 = property on="G Vel. do Motor da Válvula de Descarga" class="WFChart (strict)"("XScale.Multiplier"=w597, "XScale.NameLbl.Text"=w600) -> ()  [unwired: 2 in, 2 out]
                n417 = property on="Grafico Corrente" class="WFChart (strict)"("XScale.Multiplier"=w597, "XScale.NameLbl.Text"=w600) -> ()  [unwired: 2 in, 2 out]
                n418 = property on="Grafico Pressão" class="WFChart (strict)"("XScale.Multiplier"=w597, "XScale.NameLbl.Text"=w600) -> ()  [unwired: 2 in, 2 out]
                n419 = property on="Grafico Temperatura" class="WFChart (strict)"("XScale.Multiplier"=w597, "XScale.NameLbl.Text"=w600) -> ()  [unwired: 2 in, 2 out]
                n420 = property on="Grafico Vazão" class="WFChart (strict)"("XScale.Multiplier"=w597, "XScale.NameLbl.Text"=w600) -> ()  [unwired: 2 in, 2 out]
                n421 = property on="Grafico Vibração" class="WFChart (strict)"("XScale.Multiplier"=w597, "XScale.NameLbl.Text"=w600) -> ()  [unwired: 2 in, 2 out]
              }
              frame 3 {
                w601 = "Tempo [h]" ("X Scale.Name Label.Text")
                n422 = Divide(x=0.5 ("X Scale.Offset and Multiplier:Multiplier"), y=3600.0) -> (x/y=w604:dbl)
                n423 = property on="G Corrente RMS" class="WFChart (strict)"("XScale.Multiplier"=w604, "XScale.NameLbl.Text"=w601) -> ()  [unwired: 2 in, 2 out]
                n424 = property on="G Posição do Encoder" class="WFChart (strict)"("XScale.Multiplier"=w604, "XScale.NameLbl.Text"=w601) -> ()  [unwired: 2 in, 2 out]
                n425 = property on="G Pressão Intermed" class="WFChart (strict)"("XScale.Multiplier"=w604, "XScale.NameLbl.Text"=w601) -> ()  [unwired: 2 in, 2 out]
                n426 = property on="G Pressão de Descarga" class="WFChart (strict)"("XScale.Multiplier"=w604, "XScale.NameLbl.Text"=w601) -> ()  [unwired: 2 in, 2 out]
                n427 = property on="G Pressão de Sucção" class="WFChart (strict)"("XScale.Multiplier"=w604, "XScale.NameLbl.Text"=w601) -> ()  [unwired: 2 in, 2 out]
                n428 = property on="G Temperaturas" class="WFChart (strict)"("XScale.Multiplier"=w604, "XScale.NameLbl.Text"=w601) -> ()  [unwired: 2 in, 2 out]
                n429 = property on="G Tensão Yokogawa" class="WFChart (strict)"("XScale.Multiplier"=w604, "XScale.NameLbl.Text"=w601) -> ()  [unwired: 2 in, 2 out]
                n430 = property on="G Tensão na válvula de Sucção" class="WFChart (strict)"("XScale.Multiplier"=w604, "XScale.NameLbl.Text"=w601) -> ()  [unwired: 2 in, 2 out]
                n431 = property on="G Vazão" class="WFChart (strict)"("XScale.Multiplier"=w604, "XScale.NameLbl.Text"=w601) -> ()  [unwired: 2 in, 2 out]
                n432 = property on="G Vel. do Motor da Válvula de Descarga" class="WFChart (strict)"("XScale.Multiplier"=w604, "XScale.NameLbl.Text"=w601) -> ()  [unwired: 2 in, 2 out]
                n433 = property on="Grafico Corrente" class="WFChart (strict)"("XScale.Multiplier"=w604, "XScale.NameLbl.Text"=w601) -> ()  [unwired: 2 in, 2 out]
                n434 = property on="Grafico Pressão" class="WFChart (strict)"("XScale.Multiplier"=w604, "XScale.NameLbl.Text"=w601) -> ()  [unwired: 2 in, 2 out]
                n435 = property on="Grafico Temperatura" class="WFChart (strict)"("XScale.Multiplier"=w604, "XScale.NameLbl.Text"=w601) -> ()  [unwired: 2 in, 2 out]
                n436 = property on="Grafico Vazão" class="WFChart (strict)"("XScale.Multiplier"=w604, "XScale.NameLbl.Text"=w601) -> ()  [unwired: 2 in, 2 out]
                n437 = property on="Grafico Vibração" class="WFChart (strict)"("XScale.Multiplier"=w604, "XScale.NameLbl.Text"=w601) -> ()  [unwired: 2 in, 2 out]
              }
            }
          }
          event "Unidade Pressão": Value Change {
            n438 = event-data() -> ()  [unwired: 1 in, 6 out]
          }
        }
        n439 = call "ms2hhmmss.vi"("ms"=w543) -> ("hh:mm:ss"=→"Tempo de Ensaio":string)
        n440 = case shown="True" "Limpar Gráficos" {
          frame False {
          }
          frame True {
            w621 = T21 [] ("History Data")
            w623 = dbl[] [] ("History Data")
            w624 = T22 [] ("History Data")
            n441 = property on="G Temperaturas" class="WFChart (strict)"("History Data"=w621) -> ()  [unwired: 2 in, 2 out]
            n442 = property on="Grafico Temperatura" class="WFChart (strict)"("History Data"=w621) -> ()  [unwired: 2 in, 2 out]
            n443 = property on="G Posição do Encoder" class="WFChart (strict)"("History Data"=w624) -> ()  [unwired: 2 in, 2 out]
            n444 = property on="Grafico Vibração" class="WFChart (strict)"("History Data"=T16 []) -> ()  [unwired: 2 in, 2 out]
            n445 = property on="G Pressão de Sucção" class="WFChart (strict)"("History Data"=w624) -> ()  [unwired: 2 in, 2 out]
            n446 = property on="G Pressão de Descarga" class="WFChart (strict)"("History Data"=w624) -> ()  [unwired: 2 in, 2 out]
            n447 = property on="Grafico Pressão" class="WFChart (strict)"("History Data"=T13 []) -> ()  [unwired: 2 in, 2 out]
            n448 = property on="G Corrente RMS" class="WFChart (strict)"("History Data"=w624) -> ()  [unwired: 2 in, 2 out]
            n449 = property on="Grafico Corrente" class="WFChart (strict)"("History Data"=w624) -> ()  [unwired: 2 in, 2 out]
            n450 = property on="G Tensão Yokogawa" class="WFChart (strict)"("History Data"=w623) -> ()  [unwired: 2 in, 2 out]
            n451 = property on="G Vel. do Motor da Válvula de Descarga" class="WFChart (strict)"("History Data"=w623) -> ()  [unwired: 2 in, 2 out]
            n452 = property on="G Tensão na válvula de Sucção" class="WFChart (strict)"("History Data"=w623) -> ()  [unwired: 2 in, 2 out]
            n453 = property on="G Pressão Intermed" class="WFChart (strict)"("History Data"=w623) -> ()  [unwired: 2 in, 2 out]
            n454 = property on="Grafico Vazão" class="WFChart (strict)"("History Data"=w623) -> ()  [unwired: 2 in, 2 out]
            n455 = property on="G Vazão" class="WFChart (strict)"("History Data"=w623) -> ()  [unwired: 2 in, 2 out]
            n456 = property on="G Potência Yokogawa" class="WFChart (strict)"("History Data"=w623) -> ()  [unwired: 2 in, 2 out]
          }
        }
        n457 = Bundle("Abertura Atual da Válvula de Descarga"=w570, "Setpoint da abertura da valvula"=w569) -> (→"G Posição do Encoder":T11)  [unwired: 1 in]
        n458 = local read "Descarga [ºC]"() -> (w580:dbl)
        n459 = local read "Bobina 1 [ºC]"() -> (w535:dbl)
        n460 = local read "Ambiente [ºC]"() -> (w532:dbl)
        n461 = local read "Sucção [ºC]"() -> (w581:dbl)
        n462 = local read "RMS Superior [g]"() -> (w584:dbl)
        n463 = local read "RMS Bancada [g]"() -> (w586:dbl)
        n464 = local read "RMS Inferior [g]"() -> (w585:dbl)
        n465 = local read "Corpo [ºC]"() -> (w533:dbl)
        n466 = local read "Bobina 2 [ºC]"() -> (w536:dbl)
        n467 = local read "Reservatório [ºC]"() -> (w531:dbl)
        n468 = Bundle("Sucção [ºC]"=w581, "Descarga [ºC]"=w580, "Bobina 1 [ºC]"=w535, "Bobina 2 [ºC]"=w536, "Corpo [ºC]"=w533, "Ambiente [ºC]"=w532, "Reservatório [ºC]"=w531) -> (→"Grafico Temperatura" →"G Temperaturas":T4)  [unwired: 1 in]
        n469 = Bundle("RMS Superior [g]"=w584, "RMS Bancada [g]"=w586, "RMS Inferior [g]"=w585) -> (→"Grafico Vibração":T32)  [unwired: 1 in]
        n470 = local read "Tensão RMS [V] (WT130)"() -> (→"G Tensão Yokogawa":dbl)
        n471 = local read "Erro Fluximetro"() -> (w559:errorcluster)
        n472 = local read "Potência [W] (WT130)"() -> (→"G Potência Yokogawa":dbl)
        n473 = local read "Erro FPGA"() -> (w534:errorcluster)
        n474 = local read "Erro Pressão"() -> (w557:errorcluster)
        n475 = local read "Erro Motor"() -> (w558:errorcluster)
        n476 = local read "Erro Valv. Sucção"() -> (w556:errorcluster)
        n477 = Wait on Occurrence(1:FALSE ("ignore previous (T)"), 2:w563, 3:500 ("ms timeout (-1)")) -> (0:w565:bool)
        n478 = Not(x=w565) -> (.not. x?=w562:bool)
        n479 = Merge Errors(w559, w534, w557, w558, w556) -> (→"Error Out":errorcluster)
      }
      n480 = call <vilib>:"DAQmx Stop Task.vi"("task/channels in"=w262) -> ("task out"=w263:refnum<k21>, "error out"=w264:errorcluster)  [unwired: 13 in]
      n481 = call <vilib>:"DAQmx Stop Task.vi"("task/channels in"=w322) -> ("task out"=w321:refnum<k21>, "error out"=w320:errorcluster)  [unwired: 13 in]
      n482 = call <vilib>:"DAQmx Clear Task.vi"("task in"=w263, "error in"=w264) -> ()  [unwired: 13 in, 1 out]
      n483 = call <vilib>:"DAQmx Clear Task.vi"("task in"=w321, "error in"=w320) -> ()  [unwired: 13 in, 1 out]
      n484 = call-poly <vilib>:"DAQmx Write.vi"("task/channels in"=w277, "data"=TRUE) -> ("task out"=w278:refnum<k21>)  [unwired: 11 in, 2 out]
      n485 = call <vilib>:"DAQmx Stop Task.vi"("task/channels in"=w323) -> ("task out"=w325:refnum<k21>, "error out"=w326:errorcluster)  [unwired: 13 in]
      n486 = call <vilib>:"DAQmx Stop Task.vi"("task/channels in"=w324) -> ("task out"=w327:refnum<k21>, "error out"=w328:errorcluster)  [unwired: 13 in]
      n487 = call "Encoder End.vi"("Task Out"=w293) -> ()  [unwired: 10 in, 1 out]
      n488 = call <vilib>:"DAQmx Clear Task.vi"("task in"=w325, "error in"=w326) -> ()  [unwired: 13 in, 1 out]
      n489 = call <vilib>:"DAQmx Clear Task.vi"("task in"=w327, "error in"=w328) -> ()  [unwired: 13 in, 1 out]
      n490 = call <vilib>:"High Resolution Relative Seconds.vi"() -> ("relative seconds"=w296:dbl)
      n491 = node-c288(i64 400 ("Period")) -> (w319:T18)  [unwired: 3 in]
      n492 = timed-loop {
        tunnel: [w680] -> w283
        tunnel: w317 -> [w679]
        timing: w319 -> [_]
        timing-out: [_] -> w318
        tunnel: w296 -> [w646]
        tunnel: w292 -> [w644]
        tunnel: w288 -> [w630]
        stop <- "STOP" stop-if-true
        w635 = 99000.0 ("upper limit")
        # "Controle do setpoint da abertura\n               da válvula"
        # "Controle do motor acoplado a valvula"
        # "Controle da posição da válvula"
        # "Controle pressão Sucção"
        # "Controle Pressão e Posição"
        n493 = node-c288() -> ()  [unwired: 1 in, 1 out]
        n494 = local read "Posição Atual da Válvula de Descarga"() -> (w638:dbl)
        n495 = call <vilib>:"High Resolution Relative Seconds.vi"() -> ("relative seconds"=w647:dbl)
        n496 = local read "Descarga [bar]"() -> (w651:dbl)
        n497 = disable-structure shown="Enabled" {
          disable-tunnel: [w681 w682] -> w650
          frame Disabled {
            n498 = local read "Sucção [bar]"() -> (w681:dbl)
          }
          frame Enabled {
            n499 = local read "GE Comp S [bar]"() -> (w682:dbl)
          }
        }
        n500 = feedback #10(w646) -> (w648:dbl)
        n501 = feedback-in #10(w647) -> ()
        n502 = Subtract(x=w647, y=w648) -> (x-y=→"dt - Controle Pressão [s]":dbl)
        n503 = In Range and Coerce(upper limit=10.0, x="Tensão da válvula de sucção [V]", lower limit=0.0) -> (coerced(x)=w654:dbl)  [unwired: 1 out]
        n504 = Bundle("upper limit"=w635, "lower limit"=0.0) -> (w664:cluster{"upper limit":dbl, "lower limit":dbl})  [unwired: 1 in]
        n505 = feedback #11(TRUE ("P. Descarga Auto?")) -> (w672:bool)
        n506 = feedback-in #11("Vel. Valv. Desc. Auto?") -> ()
        n507 = Bundle("output high"=5.0, "Limite inferior - Válvula de sucção"="Limite inferior - Válvula de sucção") -> (w627:T33)  [unwired: 1 in]
        n508 = call-poly <vilib>:"PID Advanced.vi"("setpoint"="Setpoint Descarga [bar]", "output range"=w664, "auto? (T)"="P. Descarga Auto?", "manual control"="Abertura da válvula de descarga", "process variable"=w651, "PID gains"="Ganhos - Pressão de Descarga") -> ("output"=w663:dbl)  [unwired: 8 in, 1 out]
        n509 = In Range and Coerce(upper limit=w635, x=w663, lower limit=0.0) -> (coerced(x)=w662:dbl)  [unwired: 1 out]
        "Setpoint da abertura da valvula" <- w662
        n510 = Subtract(x=w638, y="Limite inferior da posição da válvula") -> (x-y=w637:dbl)
        "Abertura Atual da Válvula de Descarga" <- w637
        n511 = Not Equal?(x=w672, y="Vel. Valv. Desc. Auto?") -> (x != y?=w656:bool)
        n512 = call-poly <vilib>:"PID Advanced.vi"("setpoint"="Setpoint Sucção [bar]", "output range"=w627, "auto? (T)"="P. Sucção Auto?", "manual control"=w654, "process variable"=w650, "PID gains"="Ganhos - Pressão de Sucção") -> ("output"=→"Tensão da válvula de sucção [V]":dbl)  [unwired: 8 in, 1 out]
        n513 = case shown="True" w656 {
          tunnel: "Vel. Valv. Desc. Auto?" -> [_ w699]
          frame False {
            # "No edge"
          }
          frame True {
            # "There is an edge"
            n514 = case shown="False" w699 {
              frame False {
                # "Falling edge"
                n515 = local write "P. Descarga Auto?"(FALSE) -> ()
              }
              frame True {
                # "Rising edge"
              }
            }
          }
        }
        n516 = feedback #12(FALSE ("P. Descarga Auto?")) -> (w668:bool)
        n517 = feedback-in #12("P. Descarga Auto?") -> ()
        n518 = call-poly <vilib>:"PID Advanced.vi"("setpoint"=w662, "output range"="Limites de velocidade", "auto? (T)"="Vel. Valv. Desc. Auto?", "manual control"="Velocidade do motor de descarga", "process variable"=w637, "PID gains"="Ganhos - Posição do motor") -> ("output"=w661:dbl)  [unwired: 8 in, 1 out]
        n519 = Not Equal?(x=w668, y="P. Descarga Auto?") -> (x != y?=w667:bool)
        n520 = Unbundle("Limites de velocidade") -> ("Velocidade Máxima"=w658:dbl, "Velocidade Mínima"=w657:dbl)
        n521 = case shown="True" w667 {
          tunnel: "P. Descarga Auto?" -> [_ w697]
          frame False {
            # "No edge"
          }
          frame True {
            # "There is an edge"
            n522 = case shown="True" w697 {
              frame False {
                # "Falling edge"
              }
              frame True {
                # "Rising edge"
                n523 = local write "Vel. Valv. Desc. Auto?"(TRUE) -> ()
              }
            }
          }
        }
        n524 = In Range and Coerce(upper limit=w658, x=w661, lower limit=w657) -> (coerced(x)=w660:dbl)  [unwired: 1 out]
        "Velocidade do motor de descarga" <- w660
        n525 = To Long Integer(number=w660) -> (32bit integer=w673:i32)
        n526 = case shown="True" "STOP" {
          tunnel: w644 -> [_ w696]
          frame False {
          }
          frame True {
            n527 = Set Occurrence(w696) -> ()
            n528 = local write "STOP"(FALSE ("STOP")) -> ()
            n529 = global write "FPGA_RW_Vars.vi" "Stop"(TRUE) -> ()
          }
        }
        n530 = flat-sequence {
          tunnel: w673 -> [w685]
          tunnel: [w685] -> w634
          tunnel: w630 -> [w684]
          tunnel: [w683] -> w632
          tunnel: w679 -> [w687]
          tunnel: w634 -> [w691]
          tunnel: [w689] -> w633
          tunnel: w632 -> [w690]
          tunnel: [w690] -> w631
          tunnel: [w693] -> w680
          tunnel: w633 -> [w693]
          tunnel: w631 -> [w692]
          frame #0 {
            n531 = call <vilib>:"Acquire Semaphore.vi"("semaphore"=w684) -> ("semaphore out"=w683:T25)  [unwired: 4 in, 2 out]
          }
          frame #1 {
            n532 = call <instrlib>:"VCS Move With Velocity.vi"("error in (no error)"=errorcluster {"status"=FALSE, "code"=0, "source"=""}, "targetVelocity"=w691, "axis in"=w687) -> ("error out"=→"Erro Motor":errorcluster, "axis out"=w689:cluster{"keyHandle":u32, "nodeId":u16})  [unwired: 7 in]
          }
          frame #2 {
            n533 = call <vilib>:"Release Semaphore.vi"("semaphore"=w692) -> ()  [unwired: 5 in, 2 out]
          }
        }
        n534 = global read "FPGA_RW_Vars.vi" "Error Out"() -> (→"Erro FPGA":errorcluster)
        n535 = node-c288() -> ()  [unwired: 1 in, 1 out]
        "P. S. Auto?" <- "P. Sucção Auto?"
        "Vel. M. Auto?" <- "Vel. Valv. Desc. Auto?"
        "P. D. Auto?" <- "P. Descarga Auto?"
      }
      n536 = node-c288(w318) -> ()  [unwired: 1 out]
      n537 = call "closeCAN_EPOS+DPS.vi"("error in"=errorcluster {"status"=FALSE, "code"=0, "source"=""} ("error out"), "DPS NodeID"=w284, "ObjHandle in"=w285, "axis in"=w283) -> ()  [unwired: 7 in, 1 out]
    }
    frame #4 {
      # "Finaliza Timer segurança"
      n538 = flat-sequence {
        tunnel: w894 -> [w913]
        tunnel: [w912] -> w893
        tunnel: w893 -> [w918]
        frame #0 {
          n539 = while {
            tunnel: w913 -> [w914]
            tunnel: [w914] -> w912
            stop <- w915 stop-if-true
            n540 = global read "FPGA_RW_Vars.vi" "Reading?"() -> (w916:bool)
            n541 = Not(x=w916) -> (.not. x?=w915:bool)
          }
        }
        frame #1 {
          n542 = global read "FPGA_RW_Vars.vi" "Error Out"() -> (w919:errorcluster)
          n543 = Close Reference(reference=w918) -> ()  [unwired: 1 in, 1 out]
          n544 = local write "Erro FPGA"(w919) -> ()
          n545 = global write "FPGA_RW_Vars.vi" "Stop"(FALSE ("Stop")) -> ()
        }
      }
      n546 = flat-sequence {
        tunnel: w911 -> [w920]
        tunnel: w910 -> [w925]
        tunnel: [w924] -> w909
        tunnel: w909 -> [w929]
        frame #0 {
          # "Reset timer"
          n547 = call-poly <vilib>:"DAQmx Write.vi"("task/channels in"=w920, "data"=FALSE) -> ("task out"=w922:refnum<k21>)  [unwired: 11 in, 2 out]
          n548 = call-poly <vilib>:"DAQmx Write.vi"("task/channels in"=w925, "data"=TRUE) -> ("task out"=w924:refnum<k21>)  [unwired: 11 in, 2 out]
          n549 = call <vilib>:"DAQmx Stop Task.vi"("task/channels in"=w922) -> ("task out"=w927:refnum<k21>, "error out"=w928:errorcluster)  [unwired: 13 in]
          n550 = Wait (ms)(milliseconds to wait=u32 500) -> ()  [unwired: 1 out]
          n551 = call <vilib>:"DAQmx Clear Task.vi"("task in"=w927, "error in"=w928) -> ()  [unwired: 13 in, 1 out]
        }
        frame #1 {
          # "Clear channel"
          n552 = call-poly <vilib>:"DAQmx Write.vi"("task/channels in"=w929, "data"=FALSE) -> ("task out"=w930:refnum<k21>)  [unwired: 11 in, 2 out]
          n553 = call <vilib>:"DAQmx Stop Task.vi"("task/channels in"=w930) -> ("task out"=w932:refnum<k21>, "error out"=w933:errorcluster)  [unwired: 13 in]
          n554 = call <vilib>:"DAQmx Clear Task.vi"("task in"=w932, "error in"=w933) -> ()  [unwired: 13 in, 1 out]
        }
      }
      n555 = call <instrlib>:"Close.vi"("error in (no error)"=w905, "VISA resource name"=w906) -> ("error out"=w908:errorcluster)  [unwired: 9 in]
      n556 = call <vilib>:"Simple Error Handler.vi"("error in (no error)"=w908) -> ("error out"=→"error out":errorcluster)  [unwired: 4 in, 4 out]
      n557 = call-poly <vilib>:"DAQmx Write.vi"("task/channels in"=w896, "data"=0.0) -> ("task out"=w901:refnum<k21>)  [unwired: 11 in, 2 out]
      n558 = call-poly <vilib>:"DAQmx Write.vi"("task/channels in"=w895, "data"=0.0) -> ("task out"=w900:refnum<k21>)  [unwired: 11 in, 2 out]
      n559 = call <vilib>:"DAQmx Stop Task.vi"("task/channels in"=w901) -> ("task out"=w904:refnum<k21>, "error out"=w903:errorcluster)  [unwired: 13 in]
      n560 = call <vilib>:"DAQmx Stop Task.vi"("task/channels in"=w900) -> ("task out"=w897:refnum<k21>, "error out"=w898:errorcluster)  [unwired: 13 in]
      n561 = call <vilib>:"DAQmx Clear Task.vi"("task in"=w904, "error in"=w903) -> ()  [unwired: 13 in, 1 out]
      n562 = call <vilib>:"DAQmx Clear Task.vi"("task in"=w897, "error in"=w898) -> ()  [unwired: 13 in, 1 out]
    }
  }
